vi "(20M)art联动采集V4.9(新增双行扫描模块).vi"() -> ()   [LabVIEW 2016]
uses:
  <vilib>/Utility/file.llb/Write Delimited Spreadsheet (DBL).vi
  E:/PCI8552B/Driver/INF/Win32&Win64/amd64/PCI8552B_32.dll
  <vilib>/Instr/_visa.llb/VISA Configure Serial Port (Instr).vi
  <vilib>/Utility/file.llb/Read Delimited Spreadsheet (I64).vi
  ACTS1001_32.dll
panel:
  in  "输出宽度 3":i32=50 min=50 max=50000 step=50
  in  "输出宽度 2":i32=50 min=50 max=50000 step=50
  out "hDevice":i32=241832032
  out "采样频率":i32=10000 min=1 max=80000000 step=1
  out "使能通道总数":i32
  in  "分频数":i32=20 min=1 step=1
  in  "是否为主设备":bool caption="触发输出使能"
  in  "时钟输出":i32(ring) items=["参考时钟", "基准时钟"]
  in  "时钟输出 2":bool caption="触发输出使能"
  in  "采样时基":i32(ring) items=["内部时钟", "外部时钟"]
  in  "参考时钟":i32(ring) items=["板载时钟", "外部10M", "PXI_CLK10M", "PXIe_CLK100M"]
  in  "输出宽度":i32=50 min=50 max=50000 step=50
  in  "触发输出使能":bool
  in  "触发输出":i32(ring) items=["负向触发", "正向触发", "正负向触发"]
  in  "延时点数":i32 min=0 step=1
  in  "量程选择 3":i32(ring) items=["±5000mV"=0, "±1000mV"=2]
  in  "量程选择 2":i32(ring) items=["±5000mV"=0, "±1000mV"=2]
  in  "量程选择 1":i32(ring) items=["±5000mV"=0, "±1000mV"=2]
  in  "量程选择 0":i32(ring) items=["±5000mV"=0, "±1000mV"=2]
  in  "CH3":bool=TRUE
  in  "CH2":bool=TRUE
  in  "CH1":bool=TRUE
  in  "CH0":bool=TRUE
  in  "耦合类型1":i32(ring) items=["直流", "交流"]
  in  "耦合类型0":i32(ring) items=["直流", "交流"]
  in  "耦合类型2":i32(ring) items=["直流", "交流"]
  in  "耦合类型3":i32(ring) items=["直流", "交流"]
  in  "同步信号触发源":i32(ring) items=["TRIG0信号", "TRIG1信号", "TRIG2信号", "TRIG3信号", "TRIG4信号", "TRIG5信号", "TRIG6信号", "TRIG7信号"]
  in  "触发电平":i32=1 min=1 max=10 step=1
  in  "触发灵敏窗":i32=1 min=1 max=255 step=1
  in  "触发方向":i32(ring) items=["下降沿触发", "上升沿触发", "上升沿下降沿均触发"]
  in  "触发模式":i32(ring) items=["后触发", "硬件延时触发"]
  in  "触发源":i32(ring) items=["软件触发", "外部数字触发", "同步信号触发", "通道0触发", "通道1触发", "通道2触发", "通道3触发"]
  in  "单行？":enum32{"单行", "双行"}(radio)
  in  "色码表导入":path=path "C:/Users/H301/Desktop/art闭环扫描程序/色码表/色码表（彩色2）.txt" caption="（色码表导入）"
  out "水平进度条":u8(slide) scale=0.0..100.0
  out "x+y 3":dbl=3.0
  in  "分层图查看":bool
  in  "hDevice 2":i32
  in  "逐行扫描":bool
  in  "定位模式":bool
  in  "X终点":dbl
  in  "Y终点":dbl
  in  "高级设置":bool
  in  "Y轴回零速度":dbl=15000.0
  in  "X轴回零速度":dbl=15000.0
  in  "细分设置":dbl=8.0
  in  "等待时间":u32=40
  in  "文件保存":path=path "C:/Users/H301/Desktop/art采集实验数据" caption="保存路径"
  out "已用时（s）":dbl format="%<%H:%M:%S>t"
  out "error out":errorcluster caption="错误输出"
  in  "退出扫描(Esc)":bool
  out "毫秒计时值":u32=3586537
  out "数组":dbl[][](array[numeric])=[[58819.77200735986, 88200.32943600747]]
  out "强度图":dbl[][](graph)=[[58819.77200735986, 88200.32943600747]]
  out "judge":dbl
  out "Xloop":dbl
  out "幅频谱":dbl[](graph)
  out "时域谱":dbl[](graph)
  out "错误输出":errorcluster
  in  "启动":bool
  in  "逐点扫描":bool
  in  "X归零":bool
  in  "Y归零":bool
  in  "Y起点":dbl
  in  "Y轴速度":dbl=9000.0
  in  "X轴速度":dbl=9000.0
  out "电机状态":bool
  in  "电机端口":refnum<visa-resource-name>="COM6"
  out "Yloop":dbl=1.0
  out "X扫描范围":dbl=150.0
  out "Y扫描范围":dbl=75.0
  out "Y序":i32
  in  "X起点":dbl
  out "Y(mm)":dbl
  out "x+y 2":dbl=3.0
  in  "Y:":dbl=1.0
  in  "精度":dbl=0.001
  in  "电机急停":bool
  out "X（mm）":dbl
  out "x+y":dbl=1.0
  in  "X:":dbl=1.0
  # "实时坐标"
  # "时域谱"
  # "频域谱"
  # "归零"
  # "扫描区域"
  # "扫描步进(mm)"
  # "X:"
  # "~"
  # "Y:"
  # "~"
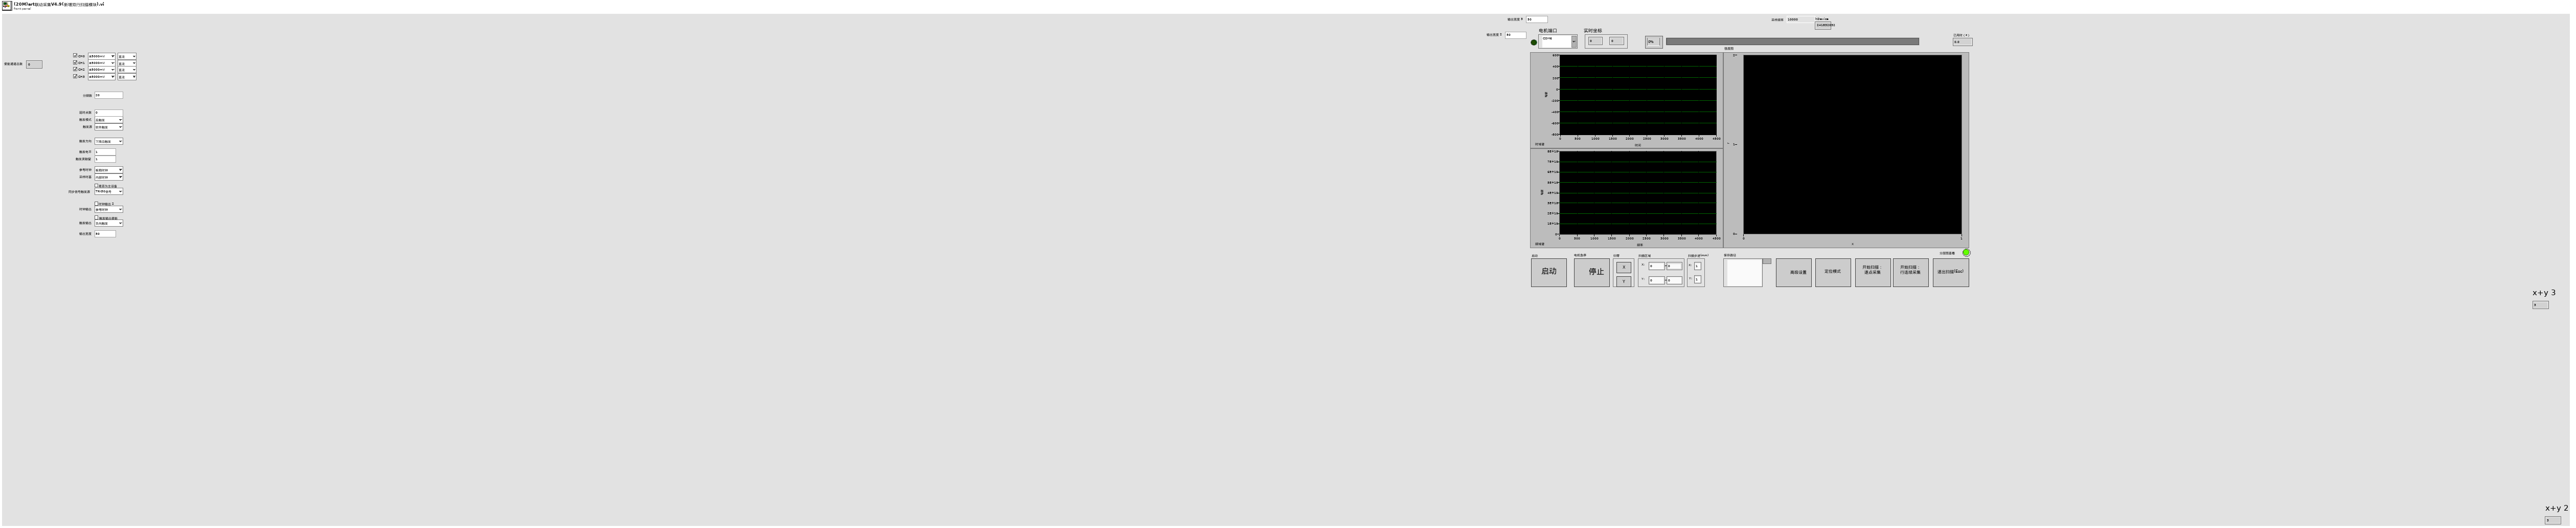
[diagram p1: front panel]
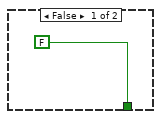
[diagram p2: hidden frame]
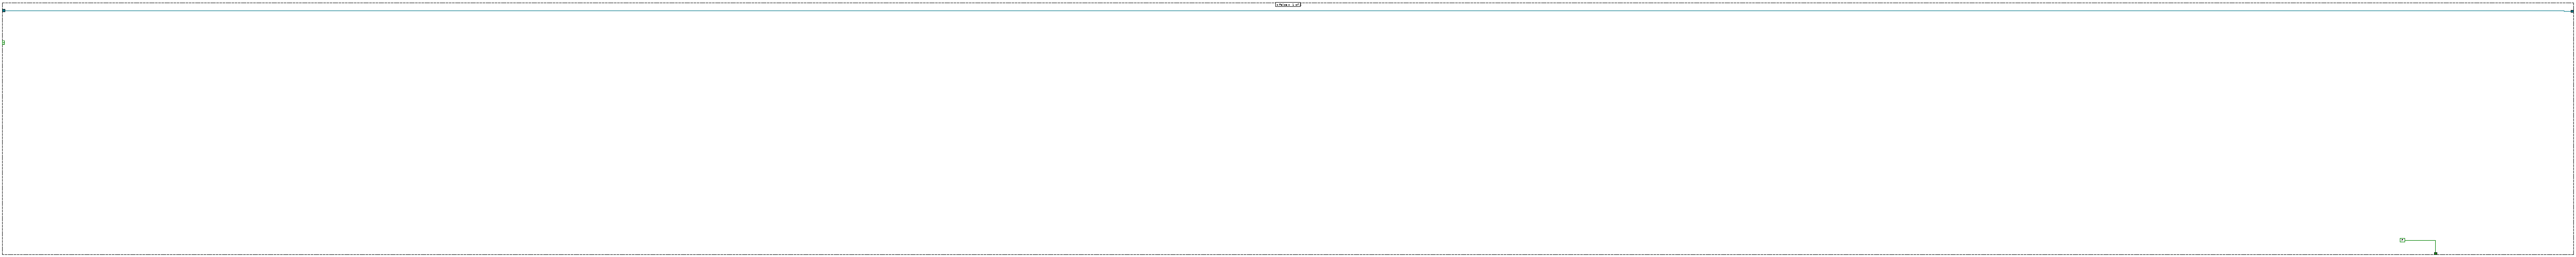
[diagram p3: hidden frame]
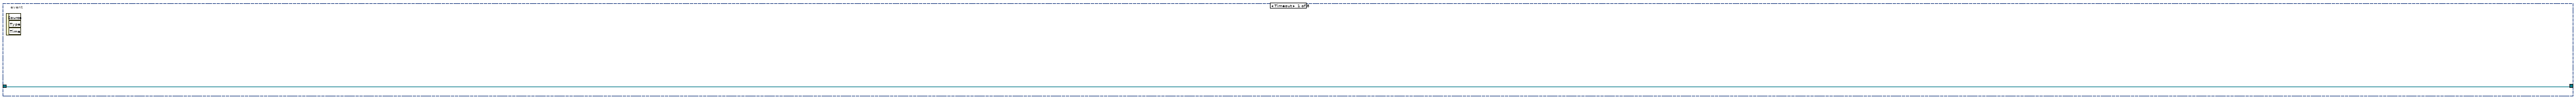
[diagram p4: hidden frame]
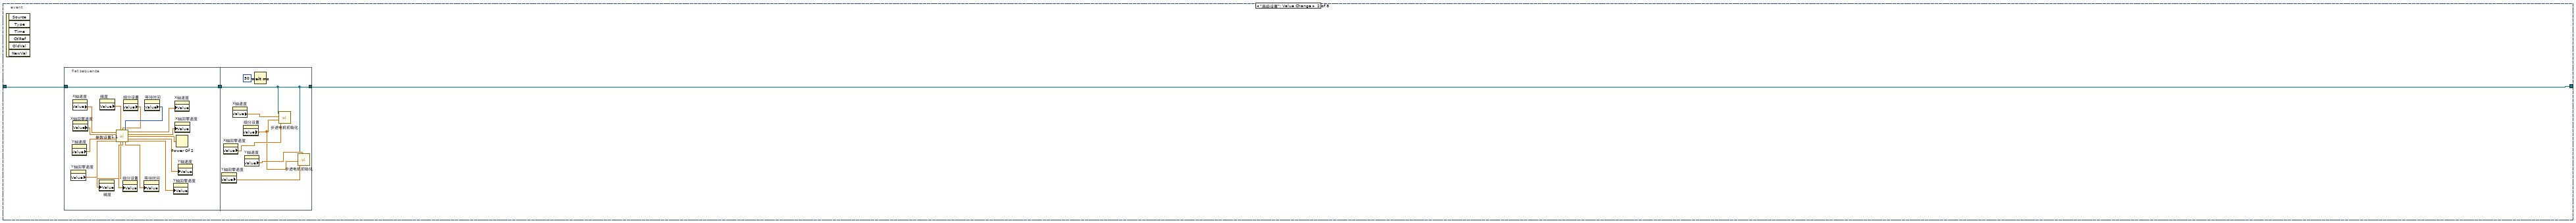
[diagram p5: hidden frame]
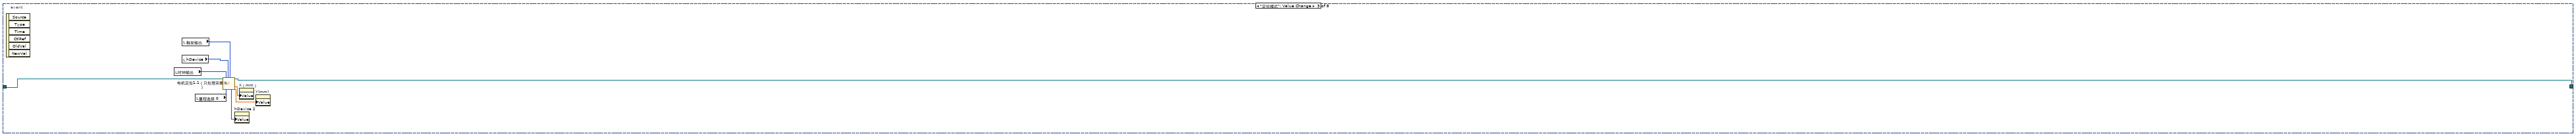
[diagram p6: hidden frame]
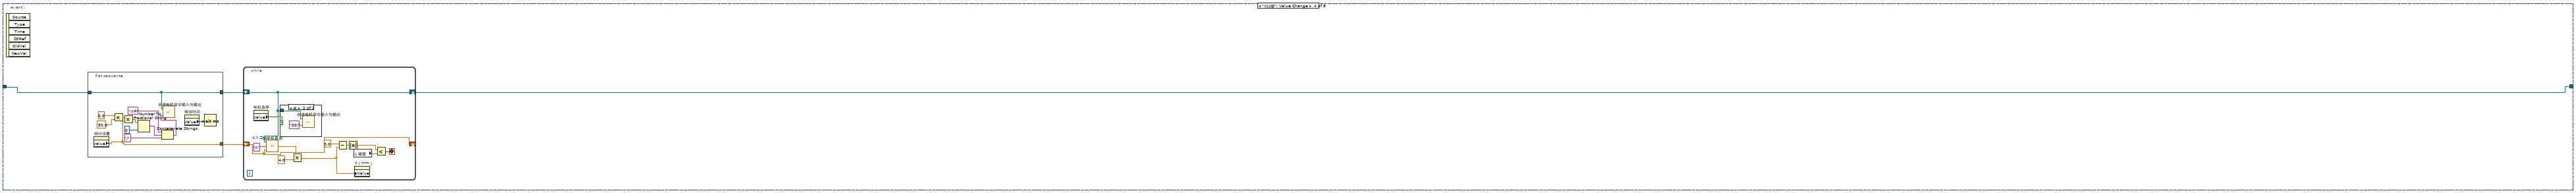
[diagram p7: hidden frame]
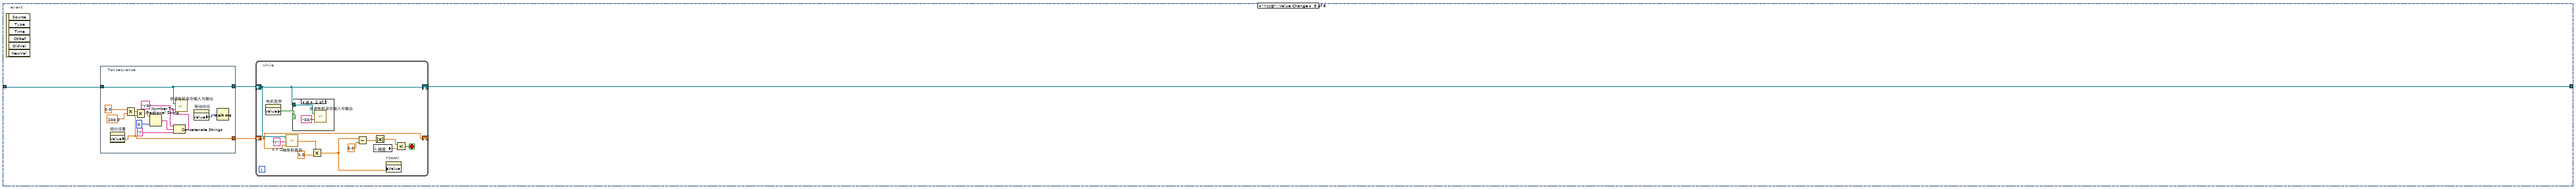
[diagram p9: hidden frame]
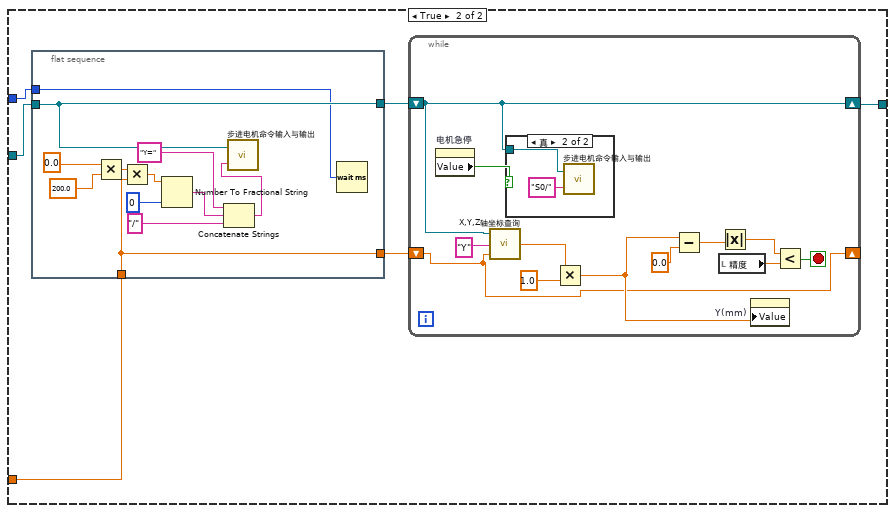
[diagram p15: hidden frame]
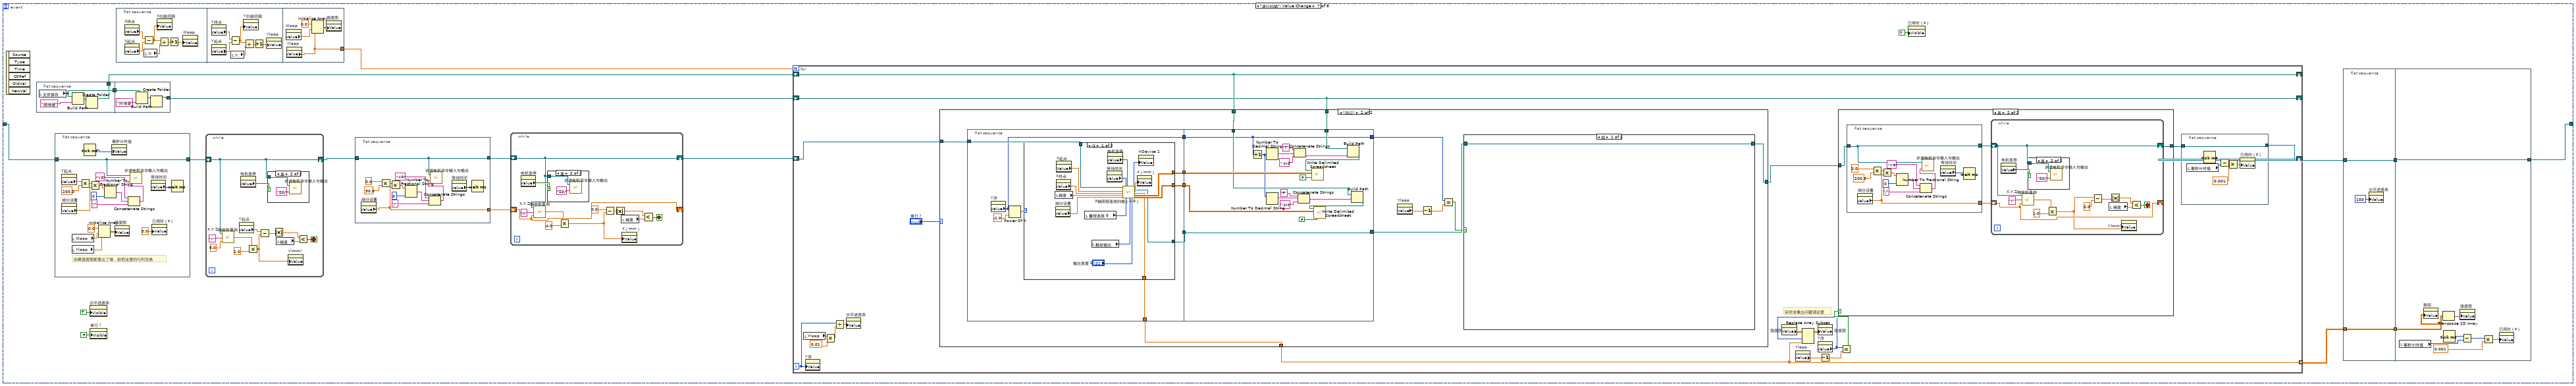
[diagram p19: hidden frame]
diagram:
  n1 = call-poly <vilib>:"Read Delimited Spreadsheet.vi"("file path (dialog if empty)"="色码表导入") -> ("first row"=w2:i64[])  [unwired: 9 in, 5 out]
  n2 = property on="强度图" class="IntGraph (严格)"("Color Table"=w2) -> ()  [unwired: 2 in, 2 out]
  n3 = property on="水平进度条" class="Slide (严格)"("Visible"=FALSE ("可见")) -> ()  [unwired: 2 in, 2 out]
  n4 = property on="单行？" class="RadioBtnsControl (严格)"("Visible"=TRUE ("可见")) -> ()  [unwired: 2 in, 2 out]
  n5 = while {
    stop <- w8 stop-if-true
    n6 = case shown="真" "启动" {
      tunnel: [FALSE ("ESC") w72] -> w8
      frame False {
      }
      frame True {
        w39 = 0 items=["边沿触发", "脉冲触发"] ("触发类型")
        w85 = u16 0 items=["无", "XON/XOFF", "RTS/CTS", "XON/XOFF & RTS/CTS", "DTR/DSR", "XON/XOFF & DTR/DSR"] ("flow control (0:none)")
        w86 = u16 10 items=["1.0"=10, "1.5"=15, "2.0"=20] ("stop bits (10: 1 bit)")
        n7 = local write item#-1(FALSE ("停止")) -> ()
        n8 = Boolean To (0,1)(Boolean="CH0") -> (0, 1=w60:i16)
        n9 = Boolean To (0,1)(Boolean="CH1") -> (0, 1=w59:i16)
        n10 = Boolean To (0,1)(Boolean="CH2") -> (0, 1=w58:i16)
        n11 = Boolean To (0,1)(Boolean="CH3") -> (0, 1=w57:i16)
        n12 = To Long Integer(number=w60) -> (32bit integer=w56:i32)
        n13 = To Long Integer(number=w59) -> (32bit integer=w55:i32)
        n14 = To Long Integer(number=w58) -> (32bit integer=w54:i32)
        n15 = To Long Integer(number=w57) -> (32bit integer=w53:i32)
        n16 = Build Array("耦合类型0", "耦合类型1", "耦合类型2", "耦合类型3") -> (w43:i32[])
        n17 = Build Array(w56, w55, w54, w53) -> (w19:i32[])
        n18 = Build Array("量程选择 0", "量程选择 1", "量程选择 2", "量程选择 3") -> (w48:i32[])
        n19 = Boolean To (0,1)(Boolean="是否为主设备") -> (0, 1=w33:i16)
        n20 = Boolean To (0,1)(Boolean="时钟输出 2") -> (0, 1=w32:i16)
        n21 = dll-call lib="ACTS1001_32.dll" fn="ACTS1001_CreateDevice"("DeviceLgcID"=0) -> ("hDevice"=w13:i32)  [unwired: 4 in, 2 out]
        n22 = Boolean To (0,1)(Boolean="触发输出使能") -> (0, 1=w31:i16)
        n23 = To Long Integer(number=w33) -> (32bit integer=w29:i32)
        n24 = To Long Integer(number=w32) -> (32bit integer=w26:i32)
        n25 = To Long Integer(number=w31) -> (32bit integer=w24:i32)
        n26 = Add Array Elements(numeric array=w19) -> (sum=→"使能通道总数":i32)
        n27 = call-poly "VISA Configure Serial Port"("VISA resource name"="电机端口", "baud rate (9600)"=u32 9600, "data bits (8)"=u16 8, "parity (0:none)"=enum16{"None", "Odd", "Even", "Mark", "Space"}."None", "stop bits (10: 1 bit)"=w86, "flow control (0:none)"=w85) -> ("VISA resource name out"=w77:refnum<visa-resource-name>, "error out"=→"error out":errorcluster)  [unwired: 1 in, 7 out]
        n28 = Build Array (concatenate)(w19, w48, w43, "分频数", "延时点数", "触发模式", "触发源", w39, "触发方向", "触发电平", "触发灵敏窗", "参考时钟", "采样时基", w29, "同步信号触发源", w26, "时钟输出", w24, "触发输出", "输出宽度") -> (w12:i32[])
        n29 = Divide(x=40000000, y="分频数") -> (x/y=→"采样频率":dbl)
        n30 = property on="细分设置" class="DigNum (严格)"() -> ("Value"=w71:dbl)  [unwired: 2 in, 2 out]
        n31 = call "步进电机初始化.vi"("回零速度"="X轴回零速度", "细分设置"=w71, "X轴速度"="X轴速度", "串口通信端口"=w77) -> ()  [unwired: 2 in, 1 out]
        n32 = call "步进电机初始化.vi"("Y轴速度"="Y轴速度", "回零速度"="Y轴回零速度", "细分设置"=w71, "串口通信端口"=w77) -> ()  [unwired: 2 in, 1 out]
        n33 = dll-call lib="ACTS1001_32.dll" fn="ACTS1001_InitDeviceAD"("hDevice"=w13, "pADPara"=w12) -> ("hDevice"=→"hDevice":i32)  [unwired: 5 in, 2 out]
        n34 = call "步进电机命令输入与输出.vi"("输入字符串"="?R/", "串口通信端口"=w77) -> ("返回字符串"=w82:string)
        n35 = String Subset(string=w82, offset (0)=0 ("偏移量(0)"), length (rest)=2 ("长度（剩余）")) -> (substring=w79:string)
        n36 = Equal?(x=w79, y="OK") -> (x = y?=w76:bool)
        "电机状态" <- w76
        n37 = case shown="真" w76 {
          tunnel: w77 -> [w92 w95]
          tunnel: [w92 w93] -> w73
          tunnel: [FALSE ("ESC") w94] -> w72
          frame False {
          }
          frame True {
            n38 = while {
              tunnel: ["退出扫描(Esc)"] -> w94
              shift-right: [w99] -> w93
              shift-left: w95 -> [w104]
              stop <- "退出扫描(Esc)" stop-if-true
              n39 = property on="水平进度条" class="Slide (严格)"("Visible"=FALSE ("可见")) -> ()  [unwired: 2 in, 2 out]
              n40 = property on="高级设置" class="Bool"("Visible"=TRUE ("可见")) -> ()  [unwired: 2 in, 2 out]
              n41 = property on="定位模式" class="Bool"("Visible"=TRUE ("可见")) -> ()  [unwired: 2 in, 2 out]
              n42 = property on="水平进度条" class="Slide (严格)"("Value"=u8 0 ("水平进度条")) -> ()  [unwired: 2 in, 2 out]
              n43 = property on="单行？" class="RadioBtnsControl (严格)"("Visible"=TRUE ("可见")) -> ()  [unwired: 2 in, 2 out]
              n44 = event shown="[5] \"逐点扫描\": 值改变" {
                selector: _ -> [_ _ _ _ _ _ _ _]
                dyn-events: _ -> [_ _ _ _ _ _ _ _]
                timeout: 1 -> [_ _ _ _ _ _ _ _]
                tunnel: w104 -> [w105 w108 w141 w145 w175 w226 w540 w905]
                tunnel: [w105 w107 w140 w143 w173 w221 w542 w904] -> w99
                event Timeout {
                  n45 = event-data() -> ()  [unwired: 1 in, 3 out]
                }
                event "高级设置": Value Change {
                  n46 = event-data() -> ()  [unwired: 1 in, 6 out]
                  n47 = flat-sequence {
                    tunnel: w108 -> [w111]
                    tunnel: [w111] -> w106
                    tunnel: [w127] -> w107
                    tunnel: w106 -> [w127]
                    frame #0 {
                      n48 = property on="Y轴回零速度" class="DigNum (严格)"() -> ("Value"=w115:dbl)  [unwired: 2 in, 2 out]
                      n49 = property on="Y轴速度" class="DigNum (严格)"() -> ("Value"=w114:dbl)  [unwired: 2 in, 2 out]
                      n50 = property on="X轴速度" class="DigNum (严格)"() -> ("Value"=w112:dbl)  [unwired: 2 in, 2 out]
                      n51 = property on="X轴回零速度" class="DigNum (严格)"() -> ("Value"=w113:dbl)  [unwired: 2 in, 2 out]
                      n52 = property on="精度" class="DigNum (严格)"() -> ("Value"=w119:dbl)  [unwired: 2 in, 2 out]
                      n53 = property on="细分设置" class="DigNum (严格)"() -> ("Value"=w120:dbl)  [unwired: 2 in, 2 out]
                      n54 = property on="等待时间" class="DigNum (严格)"() -> ("Value"=w121:u32)  [unwired: 2 in, 2 out]
                      n55 = call "参数设置1.1.vi"("X轴速度"=w112, "精度"=w119, "细分设置"=w120, "等待时间"=w121, "X轴回零速度"=w113, "Y轴速度"=w114, "Y轴回零速度"=w115) -> ("X轴速度"=w122:dbl, "X轴回零速度"=w123:dbl, "采样阶"=w109:dbl, "Y轴速度"=w124:dbl, "精度"=w116:dbl, "细分设置"=w117:dbl, "等待时间"=w118:dbl, "Y轴回零速度"=w125:dbl)  [unwired: 1 in]
                      n56 = property on="精度" class="DigNum (严格)"("Value"=w116) -> ()  [unwired: 2 in, 2 out]
                      n57 = property on="细分设置" class="DigNum (严格)"("Value"=w117) -> ()  [unwired: 2 in, 2 out]
                      n58 = property on="等待时间" class="DigNum (严格)"("Value"=w118) -> ()  [unwired: 2 in, 2 out]
                      n59 = property on="Y轴回零速度" class="DigNum (严格)"("Value"=w125) -> ()  [unwired: 2 in, 2 out]
                      n60 = property on="X轴速度" class="DigNum (严格)"("Value"=w122) -> ()  [unwired: 2 in, 2 out]
                      n61 = property on="X轴回零速度" class="DigNum (严格)"("Value"=w123) -> ()  [unwired: 2 in, 2 out]
                      n62 = Power Of 2(x=w109) -> (2^x=w110:dbl)
                      n63 = property on="Y轴速度" class="DigNum (严格)"("Value"=w124) -> ()  [unwired: 2 in, 2 out]
                    }
                    frame #1 {
                      n64 = property on="Y轴回零速度" class="DigNum (严格)"() -> ("Value"=w131:dbl)  [unwired: 2 in, 2 out]
                      n65 = property on="X轴回零速度" class="DigNum (严格)"() -> ("Value"=w130:dbl)  [unwired: 2 in, 2 out]
                      n66 = property on="X轴速度" class="DigNum (严格)"() -> ("Value"=w129:dbl)  [unwired: 2 in, 2 out]
                      n67 = property on="细分设置" class="DigNum (严格)"() -> ("Value"=w128:dbl)  [unwired: 2 in, 2 out]
                      n68 = property on="Y轴速度" class="DigNum (严格)"() -> ("Value"=w132:dbl)  [unwired: 2 in, 2 out]
                      n69 = Wait (ms)(milliseconds to wait=u32 50 ("等待时间（毫秒）")) -> ()  [unwired: 1 out]
                      n70 = call "步进电机初始化.vi"("回零速度"=w130, "细分设置"=w128, "X轴速度"=w129, "串口通信端口"=w127) -> ()  [unwired: 2 in, 1 out]
                      n71 = call "步进电机初始化.vi"("Y轴速度"=w132, "回零速度"=w131, "细分设置"=w128, "串口通信端口"=w127) -> ()  [unwired: 2 in, 1 out]
                    }
                  }
                }
                event "定位模式": Value Change {
                  n72 = event-data() -> ()  [unwired: 1 in, 6 out]
                  n73 = local read "时钟输出"() -> (w137:i32)
                  n74 = local read "触发输出"() -> (w136:i32)
                  n75 = local read "hDevice"() -> (w133:i32)
                  n76 = local read "量程选择 0"() -> (w134:i32)
                  n77 = call "电机定位1.1（只处理采集卡）.vi"("VISA I"=w141, "pulDDR2Length"=w137, "量程选择"=w134, "hDevice"=w133, "M-length"=w136) -> ("hDevice out"=w135:i32, "VISA O"=w140:refnum<visa-resource-name>, "X"=w139:dbl, "Y"=w138:dbl)  [unwired: 11 in]
                  n78 = property on="hDevice 2" class="DigNum (严格)"("Value"=w135) -> ()  [unwired: 2 in, 2 out]
                  n79 = property on="X（mm）" class="DigNum (严格)"("Value"=w139) -> ()  [unwired: 2 in, 2 out]
                  n80 = property on="Y(mm)" class="DigNum (严格)"("Value"=w138) -> ()  [unwired: 2 in, 2 out]
                }
                event "X归零": Value Change {
                  n81 = event-data() -> ()  [unwired: 1 in, 6 out]
                  n82 = flat-sequence {
                    tunnel: w145 -> [w149]
                    tunnel: [w149] -> w144
                    tunnel: [w146] -> w142
                    frame #0 {
                      n83 = property on="细分设置" class="DigNum (严格)"() -> ("Value"=w146:dbl)  [unwired: 2 in, 2 out]
                      n84 = Multiply(x=0.0, y=50.0) -> (x*y=w152:dbl)
                      n85 = Multiply(x=w152, y=w146) -> (x*y=w157:dbl)
                      n86 = Number To Fractional String(number=w157, precision (6)=i16 0 ("精度(6)")) -> (F-format string=w155:string)  [unwired: 2 out]
                      n87 = Concatenate Strings("X=" ("字符串"), w155, "/" ("字符串")) -> (w150:string)
                      n88 = call "步进电机命令输入与输出.vi"("输入字符串"=w150, "串口通信端口"=w149) -> ()  [unwired: 1 out]
                      n89 = property on="等待时间" class="DigNum (严格)"() -> ("Value"=w147:u32)  [unwired: 2 in, 2 out]
                      n90 = Wait (ms)(milliseconds to wait=w147) -> ()  [unwired: 1 out]
                    }
                  }
                  n91 = while {
                    shift-right: [w159] -> w143
                    shift-left: w144 -> [w159]
                    shift-right: [w158] -> _
                    shift-left: w142 -> [w158]
                    stop <- w165 stop-if-true
                    n92 = property on="电机急停" class="Bool (严格)"() -> ("Value"=w166:bool)  [unwired: 2 in, 2 out]
                    n93 = call "X,Y,Z轴坐标查询.vi"("细分设置"=w158, "查询坐标轴"="X", "串口通信端口"=w159) -> ("坐标(mm)"=w167:dbl)
                    n94 = case shown="真" w166 {
                      tunnel: w159 -> [_ w170]
                      frame False {
                      }
                      frame True {
                        n95 = call "步进电机命令输入与输出.vi"("输入字符串"="S0/", "串口通信端口"=w170) -> ()  [unwired: 1 out]
                      }
                    }
                    n96 = Multiply(x=w167, y=4.0 ("x")) -> (x*y=w163:dbl)
                    n97 = Subtract(x=0.0, y=w163) -> (x-y=w162:dbl)
                    n98 = Absolute Value(x=w162) -> (abs(x)=w161:dbl)
                    n99 = local read "精度"() -> (w164:dbl)
                    n100 = property on="X（mm）" class="DigNum (严格)"("Value"=w163) -> ()  [unwired: 2 in, 2 out]
                    n101 = Less?(x=w161, y=w164) -> (x < y?=w165:bool)
                  }
                }
                event "Y归零": Value Change {
                  n102 = event-data() -> ()  [unwired: 1 in, 6 out]
                  n103 = flat-sequence {
                    tunnel: w175 -> [w179]
                    tunnel: [w179] -> w174
                    tunnel: [w176] -> w172
                    frame #0 {
                      n104 = property on="细分设置" class="DigNum (严格)"() -> ("Value"=w176:dbl)  [unwired: 2 in, 2 out]
                      n105 = Multiply(x=0.0, y=200.0) -> (x*y=w182:dbl)
                      n106 = Multiply(x=w182, y=w176) -> (x*y=w187:dbl)
                      n107 = Number To Fractional String(number=w187, precision (6)=i16 0 ("精度(6)")) -> (F-format string=w185:string)  [unwired: 2 out]
                      n108 = Concatenate Strings("Y=" ("字符串"), w185, "/" ("字符串")) -> (w180:string)
                      n109 = call "步进电机命令输入与输出.vi"("输入字符串"=w180, "串口通信端口"=w179) -> ()  [unwired: 1 out]
                      n110 = property on="等待时间" class="DigNum (严格)"() -> ("Value"=w177:u32)  [unwired: 2 in, 2 out]
                      n111 = Wait (ms)(milliseconds to wait=w177) -> ()  [unwired: 1 out]
                    }
                  }
                  n112 = while {
                    shift-right: [w189] -> w173
                    shift-left: w174 -> [w189]
                    shift-right: [w188] -> _
                    shift-left: w172 -> [w188]
                    stop <- w195 stop-if-true
                    n113 = property on="电机急停" class="Bool (严格)"() -> ("Value"=w196:bool)  [unwired: 2 in, 2 out]
                    n114 = call "X,Y,Z轴坐标查询.vi"("细分设置"=w188, "查询坐标轴"="Y", "串口通信端口"=w189) -> ("坐标(mm)"=w197:dbl)
                    n115 = case shown="真" w196 {
                      tunnel: w189 -> [_ w200]
                      frame False {
                      }
                      frame True {
                        n116 = call "步进电机命令输入与输出.vi"("输入字符串"="S0/", "串口通信端口"=w200) -> ()  [unwired: 1 out]
                      }
                    }
                    n117 = Multiply(x=w197, y=1.0 ("x")) -> (x*y=w193:dbl)
                    n118 = Subtract(x=w193, y=0.0 ("x")) -> (x-y=w191:dbl)
                    n119 = local read "精度"() -> (w194:dbl)
                    n120 = Absolute Value(x=w191) -> (abs(x)=w190:dbl)
                    n121 = property on="Y(mm)" class="DigNum (严格)"("Value"=w193) -> ()  [unwired: 2 in, 2 out]
                    n122 = Less?(x=w190, y=w194) -> (x < y?=w195:bool)
                  }
                }
                event "逐点扫描": Value Change {
                  n123 = event-data() -> ()  [unwired: 1 in, 6 out]
                  n124 = flat-sequence {
                    tunnel: w226 -> [w255]
                    tunnel: [w255] -> w217
                    frame #0 {
                      # "如果强度图那里出了错，就把这里的行列互换"
                      n125 = Tick Count (ms)() -> (millisecond timer value=→"毫秒计时值":u32)
                      n126 = local read "Xloop"() -> (w250:dbl)
                      n127 = local read "Yloop"() -> (w249:dbl)
                      n128 = Multiply(x="Y起点", y=200.0) -> (x*y=w258:dbl)
                      n129 = Multiply(x=w258, y="细分设置") -> (x*y=w263:dbl)
                      n130 = Initialize Array(0.0 ("元素"), w250, w249) -> (→"强度图":dbl[][])
                      n131 = Number To Fractional String(number=w263, precision (6)=i16 0 ("精度(6)")) -> (F-format string=w261:string)  [unwired: 2 out]
                      n132 = Concatenate Strings("Y=" ("字符串"), w261, "/" ("字符串")) -> (w256:string)
                      n133 = call "步进电机命令输入与输出.vi"("输入字符串"=w256, "串口通信端口"=w255) -> ()  [unwired: 1 out]
                      n134 = property on="已用时（s）" class="DigNum (严格)"("Value"=0.0 ("已用时（s）")) -> ()  [unwired: 2 in, 2 out]
                      n135 = property on="等待时间" class="DigNum (严格)"() -> ("Value"=w247:u32)  [unwired: 2 in, 2 out]
                      n136 = Wait (ms)(milliseconds to wait=w247) -> ()  [unwired: 1 out]
                    }
                  }
                  n137 = local read "X起点"() -> (w213:dbl)
                  n138 = property on="水平进度条" class="Slide (严格)"("Visible"=TRUE ("可见")) -> ()  [unwired: 2 in, 2 out]
                  n139 = Subtract(x="X终点", y=w213) -> (x-y=w212:dbl)
                  "X扫描范围" <- w212
                  n140 = local read "X:"() -> (w220:dbl)
                  n141 = Divide(x=w212, y=w220) -> (x/y=w218:dbl)
                  n142 = Increment(x=w218) -> (x+1=→"Xloop":dbl)
                  n143 = while {
                    shift-right: [w264] -> w209
                    shift-left: w217 -> [w264]
                    stop <- w269 stop-if-true
                    n144 = call "X,Y,Z轴坐标查询.vi"("细分设置"=8.0, "查询坐标轴"="Y", "串口通信端口"=w264) -> ("坐标(mm)"=w271:dbl)
                    n145 = property on="Y起点" class="DigNum (严格)"() -> ("Value"=w273:dbl)  [unwired: 2 in, 2 out]
                    n146 = property on="电机急停" class="Bool (严格)"() -> ("Value"=w270:bool)  [unwired: 2 in, 2 out]
                    n147 = Multiply(x=w271, y=1.0 ("x")) -> (x*y=w267:dbl)
                    n148 = Subtract(x=w273, y=w267) -> (x-y=w266:dbl)
                    n149 = case shown="真" w270 {
                      tunnel: w264 -> [_ w276]
                      frame False {
                      }
                      frame True {
                        n150 = call "步进电机命令输入与输出.vi"("输入字符串"="S0/", "串口通信端口"=w276) -> ()  [unwired: 1 out]
                      }
                    }
                    n151 = Absolute Value(x=w266) -> (abs(x)=w265:dbl)
                    n152 = local read "精度"() -> (w268:dbl)
                    n153 = property on="Y(mm)" class="DigNum (严格)"("Value"=w267) -> ()  [unwired: 2 in, 2 out]
                    n154 = Less?(x=w265, y=w268) -> (x < y?=w269:bool)
                  }
                  n155 = local read "Y起点"() -> (w215:dbl)
                  n156 = Subtract(x="Y终点", y=w215) -> (x-y=w211:dbl)
                  "Y扫描范围" <- w211
                  n157 = local read "Y:"() -> (w225:dbl)
                  n158 = Divide(x=w211, y=w225) -> (x/y=w224:dbl)
                  n159 = Increment(x=w224) -> (x+1=w223:dbl)
                  "Yloop" <- w223
                  n160 = for {
                    N: w223 -> [_]
                    shift-right: [w301] -> w202
                    shift-left: w209 -> [w282]
                    tunnel: [w284] -> w222 mode=indexing
                    tunnel: w207 -> [w288]
                    tunnel: w210 -> [w287]
                    i -> [w302]
                    # "实时成像出问题调这里"
                    n161 = flat-sequence {
                      tunnel: w282 -> [w359]
                      tunnel: [w359] -> w300
                      tunnel: [w358] -> w292
                      frame #0 {
                        n162 = property on="X起点" class="DigNum (严格)"() -> ("Value"=w356:dbl)  [unwired: 2 in, 2 out]
                        n163 = property on="细分设置" class="DigNum (严格)"() -> ("Value"=w358:dbl)  [unwired: 2 in, 2 out]
                        n164 = local read "等待时间"() -> (w357:u32)
                        n165 = Multiply(x=w356, y=50.0) -> (x*y=w362:dbl)
                        n166 = Multiply(x=w362, y=w358) -> (x*y=w367:dbl)
                        n167 = Wait (ms)(milliseconds to wait=w357) -> ()  [unwired: 1 out]
                        n168 = Number To Fractional String(number=w367, precision (6)=i16 0 ("精度(6)")) -> (F-format string=w365:string)  [unwired: 2 out]
                        n169 = Concatenate Strings("X=" ("字符串"), w365, "/" ("字符串")) -> (w360:string)
                        n170 = call "步进电机命令输入与输出.vi"("输入字符串"=w360, "串口通信端口"=w359) -> ()  [unwired: 1 out]
                      }
                    }
                    n171 = while {
                      shift-right: [w369] -> w280
                      shift-left: w300 -> [w369]
                      shift-right: [w368] -> _
                      shift-left: w292 -> [w368]
                      stop <- w374 stop-if-true
                      n172 = property on="电机急停" class="Bool (严格)"() -> ("Value"=w375:bool)  [unwired: 2 in, 2 out]
                      n173 = case shown="真" w375 {
                        tunnel: w369 -> [_ w380]
                        frame False {
                        }
                        frame True {
                          n174 = call "步进电机命令输入与输出.vi"("输入字符串"="S0/", "串口通信端口"=w380) -> ()  [unwired: 1 out]
                        }
                      }
                      n175 = call "X,Y,Z轴坐标查询.vi"("细分设置"=w368, "查询坐标轴"="X", "串口通信端口"=w369) -> ("坐标(mm)"=w376:dbl)
                      n176 = Multiply(x=w376, y=4.0 ("x")) -> (x*y=w372:dbl)
                      n177 = property on="X起点" class="DigNum (严格)"() -> ("Value"=w378:dbl)  [unwired: 2 in, 2 out]
                      n178 = Subtract(x=w378, y=w372) -> (x-y=w371:dbl)
                      n179 = Absolute Value(x=w371) -> (abs(x)=w370:dbl)
                      n180 = local read "精度"() -> (w373:dbl)
                      n181 = property on="X（mm）" class="DigNum (严格)"("Value"=w372) -> ()  [unwired: 2 in, 2 out]
                      n182 = Less?(x=w370, y=w373) -> (x < y?=w374:bool)
                    }
                    n183 = local read "Xloop"() -> (w293:dbl)
                    n184 = for {
                      N: w293 -> [_]
                      shift-right: [w463] -> w281
                      shift-left: w280 -> [w459]
                      tunnel: [w462] -> w299 mode=indexing
                      tunnel: [w461] -> w298 mode=indexing
                      tunnel: [w460] -> w284 mode=indexing
                      i -> [w451]
                      n185 = flat-sequence {
                        tunnel: w459 -> [w468]
                        tunnel: [w467] -> w464
                        tunnel: w451 -> [w465]
                        tunnel: [w526] -> w463
                        tunnel: w464 -> [w526]
                        tunnel: [w525] -> w462
                        tunnel: [w524] -> w461
                        tunnel: [w522] -> w460
                        frame #0 {
                          n186 = Equal To 0?(x=w465) -> (x = 0?=w466:bool)
                          n187 = case shown="假" w466 {
                            tunnel: w468 -> [w471 w506]
                            tunnel: [w470 w506] -> w467
                            frame False {
                              n188 = flat-sequence {
                                tunnel: w471 -> [w481]
                                tunnel: [w481] -> w472
                                tunnel: [w473] -> w469
                                frame #0 {
                                n189 = local read "X:"() -> (w475:dbl)
                                n190 = Multiply(x=w475, y=1.0 ("x")) -> (x*y=w480:dbl)
                                n191 = property on="等待时间" class="DigNum (严格)"() -> ("Value"=w474:u32)  [unwired: 2 in, 2 out]
                                n192 = property on="细分设置" class="DigNum (严格)"() -> ("Value"=w473:dbl)  [unwired: 2 in, 2 out]
                                n193 = call "X,Y,Z轴坐标查询.vi"("细分设置"=w473, "查询坐标轴"="X", "串口通信端口"=w481) -> ("坐标(mm)"=w477:dbl)
                                n194 = Multiply(x=4.0, y=w477) -> (x*y=w476:dbl)
                                n195 = Add(x=w476, y=w480) -> (x+y=w483:dbl)
                                "x+y" <- w483
                                n196 = Multiply(x=w483, y=50.0) -> (x*y=w486:dbl)
                                n197 = Multiply(x=w486, y=w473) -> (x*y=w491:dbl)
                                n198 = Number To Fractional String(number=w491, precision (6)=i16 0 ("精度(6)")) -> (F-format string=w489:string)  [unwired: 2 out]
                                n199 = Concatenate Strings("X=" ("字符串"), w489, "/" ("字符串")) -> (w484:string)
                                n200 = call "步进电机命令输入与输出.vi"("输入字符串"=w484, "串口通信端口"=w481) -> ()  [unwired: 1 out]
                                n201 = Wait (ms)(milliseconds to wait=w474) -> ()  [unwired: 1 out]
                                }
                              }
                              n202 = while {
                                shift-right: [w501] -> w470
                                shift-left: w472 -> [w501]
                                shift-right: [w492] -> _
                                shift-left: w469 -> [w492]
                                stop <- w500 stop-if-true
                                n203 = property on="电机急停" class="Bool (严格)"() -> ("Value"=w498:bool)  [unwired: 2 in, 2 out]
                                n204 = local read "x+y"() -> (w502:dbl)
                                n205 = case shown="真" w498 {
                                tunnel: w501 -> [_ w504]
                                frame False {
                                }
                                frame True {
                                n206 = call "步进电机命令输入与输出.vi"("输入字符串"="S0/", "串口通信端口"=w504) -> ()  [unwired: 1 out]
                                }
                                }
                                n207 = call "X,Y,Z轴坐标查询.vi"("细分设置"=w492, "查询坐标轴"="X", "串口通信端口"=w501) -> ("坐标(mm)"=w496:dbl)
                                n208 = Multiply(x=4.0, y=w496) -> (x*y=w495:dbl)
                                n209 = Subtract(x=w502, y=w495) -> (x-y=w494:dbl)
                                n210 = property on="X（mm）" class="DigNum (严格)"("Value"=w495) -> ()  [unwired: 2 in, 2 out]
                                n211 = Absolute Value(x=w494) -> (abs(x)=w493:dbl)
                                n212 = local read "精度"() -> (w497:dbl)
                                n213 = Less?(x=w493, y=w497) -> (x < y?=w500:bool)
                              }
                            }
                            frame True {
                            }
                          }
                        }
                        frame #1 {
                          n214 = local read item#-1() -> (w520)
                          n215 = local read item#-1() -> (w521)
                          n216 = call "AD（V3.2）.vi"("M-length"=w520, 11:w521) -> ("幅频谱"=w524:dbl[], "时域谱"=w525:dbl[], "hDevice out"=w508:i32, "N-length"=w509:dbl, "hDevice"=w507:i32)  [unwired: 5 in]
                          "时域谱" <- w525
                          "幅频谱" <- w524
                          n217 = Subtract(x=w509, y=w520) -> (x-y=w518:dbl)
                          n218 = Multiply(x=w518, y=0.25) -> (x*y=w511:dbl)
                          n219 = Multiply(x=w511, y=0.442) -> (x*y=w513:dbl)
                          n220 = Multiply(x=w511, y=0.058) -> (x*y=w515:dbl)
                          n221 = Round Toward -Infinity(1:w513) -> (0:w510:dbl)
                          n222 = Round Toward -Infinity(1:w515) -> (0:w514:dbl)
                          n223 = Increment(x=w510) -> (x+1=w517:dbl)
                          n224 = property on="hDevice 2" class="DigNum (严格)"("Value"=w508) -> ()  [unwired: 2 in, 2 out]
                          n225 = Array Subset(array=w524, index=w514, length=w517) -> (w523:dbl[])
                          n226 = Array Max & Min(array=w523) -> (max value=w522:dbl)  [unwired: 3 out]
                        }
                      }
                      n227 = local read "Y序"() -> (w453:i32)
                      n228 = local read "Xloop"() -> (w454:dbl)
                      n229 = Multiply(x=w453, y=w454) -> (x*y=w452:dbl)
                      n230 = Add(x=w451, y=w452) -> (x+y=w450:dbl)
                      n231 = Multiply(x=w450, y=100.0) -> (x*y=w448:dbl)
                      n232 = local read "Xloop"() -> (w458:dbl)
                      n233 = local read "Yloop"() -> (w457:dbl)
                      n234 = Multiply(x=w457, y=w458) -> (x*y=w456:dbl)
                      n235 = Divide(x=w448, y=w456) -> (x/y=→"水平进度条":dbl)
                    }
                    n236 = flat-sequence {
                      tunnel: w298 -> [w342]
                      tunnel: w299 -> [w350]
                      tunnel: w281 -> [w354]
                      tunnel: [w354] -> w294
                      tunnel: w288 -> [w337]
                      tunnel: w287 -> [w336]
                      frame #0 {
                        n237 = local read "Y序"() -> (w338:i32)
                        n238 = Increment(x=w338) -> (x+1=w339:i32)
                        n239 = Number To Decimal String(number=w339) -> (decimal integer string=w348:string)  [unwired: 1 in]
                        n240 = Number To Decimal String(number=w339) -> (decimal integer string=w347:string)  [unwired: 1 in]
                        n241 = Concatenate Strings("T" ("字符串"), w348, ".txt" ("字符串")) -> (w351:string)
                        n242 = Concatenate Strings("F" ("字符串"), w347, ".txt" ("字符串")) -> (w345:string)
                        n243 = Build Path(base path=w337, name or relative path=w351) -> (appended path=w353:path)
                        n244 = call-poly <vilib>:"Write Delimited Spreadsheet.vi"("file path (dialog if empty)"=w353, "2D data"=w350, "transpose? (no:F)"=FALSE) -> ()  [unwired: 11 in, 2 out]
                        n245 = Build Path(base path=w336, name or relative path=w345) -> (appended path=w343:path)
                        n246 = call-poly <vilib>:"Write Delimited Spreadsheet.vi"("file path (dialog if empty)"=w343, "2D data"=w342, "transpose? (no:F)"=FALSE) -> ()  [unwired: 11 in, 2 out]
                        "judge" <- 1.0
                      }
                    }
                    n247 = flat-sequence {
                      tunnel: w294 -> [w313]
                      tunnel: [w313] -> w295
                      tunnel: [w311] -> w291
                      frame #0 {
                        n248 = property on="细分设置" class="DigNum (严格)"() -> ("Value"=w311:dbl)  [unwired: 2 in, 2 out]
                        n249 = property on="等待时间" class="DigNum (严格)"() -> ("Value"=w310:u32)  [unwired: 2 in, 2 out]
                        n250 = Multiply(x=0.0, y=50.0) -> (x*y=w316:dbl)
                        n251 = Multiply(x=w316, y=w311) -> (x*y=w321:dbl)
                        n252 = Wait (ms)(milliseconds to wait=w310) -> ()  [unwired: 1 out]
                        n253 = Number To Fractional String(number=w321, precision (6)=i16 0 ("精度(6)")) -> (F-format string=w319:string)  [unwired: 2 out]
                        n254 = Concatenate Strings("X=" ("字符串"), w319, "/" ("字符串")) -> (w314:string)
                        n255 = call "步进电机命令输入与输出.vi"("输入字符串"=w314, "串口通信端口"=w313) -> ()  [unwired: 1 out]
                      }
                    }
                    n256 = while {
                      shift-right: [w323] -> w279
                      shift-left: w295 -> [w323]
                      shift-right: [w322] -> _
                      shift-left: w291 -> [w322]
                      stop <- w329 stop-if-true
                      n257 = property on="电机急停" class="Bool (严格)"() -> ("Value"=w330:bool)  [unwired: 2 in, 2 out]
                      n258 = call "X,Y,Z轴坐标查询.vi"("细分设置"=w322, "查询坐标轴"="X", "串口通信端口"=w323) -> ("坐标(mm)"=w331:dbl)
                      n259 = case shown="真" w330 {
                        tunnel: w323 -> [_ w334]
                        frame False {
                        }
                        frame True {
                          n260 = call "步进电机命令输入与输出.vi"("输入字符串"="S0/", "串口通信端口"=w334) -> ()  [unwired: 1 out]
                        }
                      }
                      n261 = Multiply(x=w331, y=4.0 ("x")) -> (x*y=w327:dbl)
                      n262 = Subtract(x=0.0, y=w327) -> (x-y=w326:dbl)
                      n263 = Absolute Value(x=w326) -> (abs(x)=w325:dbl)
                      n264 = local read "精度"() -> (w328:dbl)
                      n265 = property on="X（mm）" class="DigNum (严格)"("Value"=w327) -> ()  [unwired: 2 in, 2 out]
                      n266 = Less?(x=w325, y=w328) -> (x < y?=w329:bool)
                    }
                    n267 = property on="强度图" class="IntGraph (严格)"() -> ("Value"=w285:dbl[][])  [unwired: 2 in, 2 out]
                    n268 = local read "Yloop"() -> (w296:dbl)
                    n269 = Decrement(x=w296) -> (x-1=w297:dbl)
                    n270 = local read "Y序"() -> (w283:i32)
                    n271 = Replace Array Subset(array=w285, new element=w284, index (col)=w283) -> (w286:dbl[][])  [unwired: 1 in]
                    n272 = property on="强度图" class="IntGraph (严格)"("Value"=w286) -> ()  [unwired: 2 in, 2 out]
                    n273 = Equal?(x=w283, y=w297) -> (x = y?=w303:bool)
                    n274 = Increment(x=w283) -> ()  [unwired: 1 out]
                    n275 = flat-sequence {
                      tunnel: w279 -> [w309]
                      tunnel: [w309] -> w278
                      frame #0 {
                        n276 = local read "毫秒计时值"() -> (w304:u32)
                        n277 = Tick Count (ms)() -> (millisecond timer value=w308:u32)
                        n278 = Subtract(x=w308, y=w304) -> (x-y=w305:u32)
                        n279 = Multiply(x=w305, y=0.001) -> (x*y=→"已用时（s）":dbl)
                      }
                    }
                    n280 = property on="细分设置" class="DigNum (严格)"() -> ("Value"=w289:dbl)  [unwired: 2 in, 2 out]
                    n281 = property on="等待时间" class="DigNum (严格)"() -> ("Value"=w290:u32)  [unwired: 2 in, 2 out]
                    n282 = case shown="假" w303 {
                      tunnel: w278 -> [w387 w419]
                      tunnel: [w385 w420] -> w301
                      tunnel: w290 -> [w383 w417]
                      tunnel: w289 -> [w382 w416]
                      frame False {
                        n283 = flat-sequence {
                          tunnel: w387 -> [w391]
                          tunnel: [w391] -> w386
                          tunnel: [w389] -> w384
                          tunnel: w383 -> [w390]
                          tunnel: w382 -> [w389]
                          frame #0 {
                            n284 = call "X,Y,Z轴坐标查询.vi"("细分设置"=w389, "查询坐标轴"="Y", "串口通信端口"=w391) -> ("坐标(mm)"=w392:dbl)
                            n285 = property on="Y:" class="DigNum (严格)"() -> ("Value"=w388:dbl)  [unwired: 2 in, 2 out]
                            n286 = Add(x=w392, y=w388) -> (x+y=w394:dbl)
                            "x+y 2" <- w394
                            n287 = Multiply(x=w394, y=200.0) -> (x*y=w398:dbl)
                            n288 = Multiply(x=w398, y=8.0 ("细分设置")) -> (x*y=w403:dbl)
                            n289 = Number To Fractional String(number=w403, precision (6)=i16 0 ("精度(6)")) -> (F-format string=w401:string)  [unwired: 2 out]
                            n290 = Concatenate Strings("Y=" ("字符串"), w401, "/" ("字符串")) -> (w396:string)
                            n291 = call "步进电机命令输入与输出.vi"("输入字符串"=w396, "串口通信端口"=w391) -> ()  [unwired: 1 out]
                            n292 = Wait (ms)(milliseconds to wait=w390) -> ()  [unwired: 1 out]
                          }
                        }
                        n293 = while {
                          shift-right: [w405] -> w385
                          shift-left: w386 -> [w405]
                          shift-right: [w404] -> _
                          shift-left: w384 -> [w404]
                          stop <- w411 stop-if-true
                          n294 = call "X,Y,Z轴坐标查询.vi"("细分设置"=w404, "查询坐标轴"="Y", "串口通信端口"=w405) -> ("坐标(mm)"=w409:dbl)
                          n295 = local read "x+y 2"() -> (w412:dbl)
                          n296 = property on="电机急停" class="Bool (严格)"() -> ("Value"=w408:bool)  [unwired: 2 in, 2 out]
                          n297 = property on="Y(mm)" class="DigNum (严格)"("Value"=w409) -> ()  [unwired: 2 in, 2 out]
                          n298 = case shown="真" w408 {
                            tunnel: w405 -> [_ w414]
                            frame False {
                            }
                            frame True {
                              n299 = call "步进电机命令输入与输出.vi"("输入字符串"="S0/", "串口通信端口"=w414) -> ()  [unwired: 1 out]
                            }
                          }
                          n300 = Subtract(x=w412, y=w409) -> (x-y=w407:dbl)
                          n301 = Absolute Value(x=w407) -> (abs(x)=w406:dbl)
                          n302 = local read "精度"() -> (w410:dbl)
                          n303 = Less?(x=w406, y=w410) -> (x < y?=w411:bool)
                        }
                      }
                      frame True {
                        n304 = flat-sequence {
                          tunnel: [w424] -> _
                          tunnel: [w424] -> w421
                          tunnel: w419 -> [w424]
                          tunnel: [w422] -> w418
                          tunnel: w417 -> [w423]
                          tunnel: w416 -> [w422]
                          frame #0 {
                            n305 = Multiply(x=0.0, y=200.0) -> (x*y=w428:dbl)
                            n306 = Multiply(x=w428, y=w422) -> (x*y=w433:dbl)
                            n307 = Number To Fractional String(number=w433, precision (6)=i16 0 ("精度(6)")) -> (F-format string=w431:string)  [unwired: 2 out]
                            n308 = Concatenate Strings("Y=" ("字符串"), w431, "/" ("字符串")) -> (w426:string)
                            n309 = call "步进电机命令输入与输出.vi"("输入字符串"=w426, "串口通信端口"=w424) -> ()  [unwired: 1 out]
                            n310 = Wait (ms)(milliseconds to wait=w423) -> ()  [unwired: 1 out]
                          }
                        }
                        n311 = while {
                          shift-right: [w435] -> w420
                          shift-left: w421 -> [w435]
                          shift-right: [w434] -> _
                          shift-left: w418 -> [w434]
                          stop <- w441 stop-if-true
                          n312 = property on="电机急停" class="Bool (严格)"() -> ("Value"=w442:bool)  [unwired: 2 in, 2 out]
                          n313 = call "X,Y,Z轴坐标查询.vi"("细分设置"=w434, "查询坐标轴"="Y", "串口通信端口"=w435) -> ("坐标(mm)"=w443:dbl)
                          n314 = case shown="真" w442 {
                            tunnel: w435 -> [_ w446]
                            frame False {
                            }
                            frame True {
                              n315 = call "步进电机命令输入与输出.vi"("输入字符串"="S0/", "串口通信端口"=w446) -> ()  [unwired: 1 out]
                            }
                          }
                          n316 = Multiply(x=w443, y=1.0 ("x")) -> (x*y=w439:dbl)
                          n317 = Subtract(x=w439, y=0.0 ("x")) -> (x-y=w437:dbl)
                          n318 = local read "精度"() -> (w440:dbl)
                          n319 = Absolute Value(x=w437) -> (abs(x)=w436:dbl)
                          n320 = property on="Y(mm)" class="DigNum (严格)"("Value"=w439) -> ()  [unwired: 2 in, 2 out]
                          n321 = Less?(x=w436, y=w440) -> (x < y?=w441:bool)
                        }
                      }
                    }
                    "Y序" <- w302
                  }
                  n322 = property on="已用时（s）" class="DigNum (严格)"("Visible"=TRUE ("可见")) -> ()  [unwired: 2 in, 2 out]
                  n323 = flat-sequence {
                    tunnel: [w227] -> w210
                    tunnel: ["文件保存"] -> w208
                    tunnel: w208 -> [w232]
                    tunnel: [w231] -> w207
                    frame #0 {
                      n324 = Build Path(base path="文件保存", name or relative path="频域谱" ("名称或相对路径")) -> (appended path=w230:path)
                      n325 = Create Folder(path (use dialog)=w230) -> (created path=w227:path)  [unwired: 2 in, 2 out]
                    }
                    frame #1 {
                      n326 = Build Path(base path=w232, name or relative path="时域谱" ("名称或相对路径")) -> (appended path=w233:path)
                      n327 = Create Folder(path (use dialog)=w233) -> (created path=w231:path)  [unwired: 2 in, 2 out]
                    }
                  }
                  n328 = flat-sequence {
                    tunnel: w222 -> [w237]
                    tunnel: [w235] -> _
                    tunnel: [w235] -> w204
                    tunnel: [w237] -> w203
                    tunnel: w202 -> [w235]
                    tunnel: [w238] -> w221
                    tunnel: w204 -> [w238]
                    tunnel: w203 -> [w241]
                    frame #0 {
                      n329 = property on="水平进度条" class="Slide (严格)"("Value"=u8 100 ("水平进度条")) -> ()  [unwired: 2 in, 2 out]
                    }
                    frame #1 {
                      n330 = local read "毫秒计时值"() -> (w240:u32)
                      n331 = Tick Count (ms)() -> (millisecond timer value=w245:u32)
                      n332 = Transpose 2D Array(2D array=w241) -> (transposed array=w242:dbl[][])
                      n333 = Subtract(x=w245, y=w240) -> (x-y=w243:u32)
                      n334 = property on="强度图" class="IntGraph (严格)"("Value"=w242) -> ()  [unwired: 2 in, 2 out]
                      n335 = Multiply(x=w243, y=0.001) -> (x*y=w239:dbl)
                      n336 = property on="已用时（s）" class="DigNum (严格)"("Value"=w239) -> ()  [unwired: 2 in, 2 out]
                      "数组" <- w241
                    }
                  }
                }
                event "逐行扫描": Value Change {
                  n337 = event-data() -> ()  [unwired: 1 in, 6 out]
                  n338 = flat-sequence {
                    tunnel: [w631] -> w544
                    tunnel: [w630] -> w541
                    tunnel: w544 -> [w635]
                    tunnel: [w634] -> w543
                    frame #0 {
                      n339 = local read "文件保存"() -> (w631:path)
                      n340 = Build Path(base path=w631, name or relative path="频域谱" ("名称或相对路径")) -> (appended path=w633:path)
                      n341 = Create Folder(path (use dialog)=w633) -> (created path=w630:path)  [unwired: 2 in, 2 out]
                    }
                    frame #1 {
                      n342 = Build Path(base path=w635, name or relative path="时域谱" ("名称或相对路径")) -> (appended path=w636:path)
                      n343 = Create Folder(path (use dialog)=w636) -> (created path=w634:path)  [unwired: 2 in, 2 out]
                    }
                  }
                  n344 = flat-sequence {
                    tunnel: [w588] -> w539
                    tunnel: w540 -> [w588]
                    frame #0 {
                      # "如果强度图那里出了错，就把这里的行列互换"
                      n345 = property on="Y起点" class="DigNum (严格)"() -> ("Value"=w591:dbl)  [unwired: 2 in, 2 out]
                      n346 = property on="细分设置" class="DigNum (严格)"() -> ("Value"=w589:dbl)  [unwired: 2 in, 2 out]
                      n347 = local read "Xloop"() -> (w595:dbl)
                      n348 = local read "Yloop"() -> (w594:dbl)
                      n349 = Multiply(x=w591, y=200.0) -> (x*y=w599:dbl)
                      n350 = Tick Count (ms)() -> (millisecond timer value=w592:u32)
                      n351 = Multiply(x=w599, y=w589) -> (x*y=w604:dbl)
                      n352 = Initialize Array(0.0 ("元素"), w595, w594) -> (w590:dbl[][])
                      n353 = Number To Fractional String(number=w604, precision (6)=i16 0 ("精度(6)")) -> (F-format string=w602:string)  [unwired: 2 out]
                      n354 = property on="毫秒计时值" class="DigNum (严格)"("Value"=w592) -> ()  [unwired: 2 in, 2 out]
                      n355 = property on="强度图" class="IntGraph (严格)"("Value"=w590) -> ()  [unwired: 2 in, 2 out]
                      n356 = Concatenate Strings("Y=" ("字符串"), w602, "/" ("字符串")) -> (w597:string)
                      n357 = call "步进电机命令输入与输出.vi"("输入字符串"=w597, "串口通信端口"=w588) -> ()  [unwired: 1 out]
                      n358 = property on="等待时间" class="DigNum (严格)"() -> ("Value"=w593:u32)  [unwired: 2 in, 2 out]
                      n359 = property on="已用时（s）" class="DigNum (严格)"("Value"=0.0 ("已用时（s）")) -> ()  [unwired: 2 in, 2 out]
                      n360 = Wait (ms)(milliseconds to wait=w593) -> ()  [unwired: 1 out]
                    }
                  }
                  n361 = property on="水平进度条" class="Slide (严格)"("Visible"=TRUE ("可见")) -> ()  [unwired: 2 in, 2 out]
                  n362 = property on="单行？" class="RadioBtnsControl (严格)"("Visible"=FALSE ("可见")) -> ()  [unwired: 2 in, 2 out]
                  n363 = flat-sequence {
                    tunnel: [w583] -> w538
                    frame #0 {
                      n364 = property on="X终点" class="DigNum (严格)"() -> ("Value"=w572:dbl)  [unwired: 2 in, 2 out]
                      n365 = property on="X起点" class="DigNum (严格)"() -> ("Value"=w571:dbl)  [unwired: 2 in, 2 out]
                      n366 = Subtract(x=w572, y=w571) -> (x-y=w576:dbl)
                      n367 = local read "X:"() -> (w575:dbl)
                      n368 = property on="X扫描范围" class="DigNum (严格)"("Value"=w576) -> ()  [unwired: 2 in, 2 out]
                      n369 = Divide(x=w576, y=w575) -> (x/y=w574:dbl)
                      n370 = Increment(x=w574) -> (x+1=w573:dbl)
                      n371 = property on="Xloop" class="DigNum (严格)"("Value"=w573) -> ()  [unwired: 2 in, 2 out]
                    }
                    frame #1 {
                      n372 = property on="Y终点" class="DigNum (严格)"() -> ("Value"=w578:dbl)  [unwired: 2 in, 2 out]
                      n373 = property on="Y起点" class="DigNum (严格)"() -> ("Value"=w577:dbl)  [unwired: 2 in, 2 out]
                      n374 = Subtract(x=w578, y=w577) -> (x-y=w581:dbl)
                      n375 = local read "Y:"() -> (w580:dbl)
                      n376 = property on="Y扫描范围" class="DigNum (严格)"("Value"=w581) -> ()  [unwired: 2 in, 2 out]
                      n377 = Divide(x=w581, y=w580) -> (x/y=w582:dbl)
                      n378 = Increment(x=w582) -> (x+1=w579:dbl)
                      n379 = property on="Yloop" class="DigNum (严格)"("Value"=w579) -> ()  [unwired: 2 in, 2 out]
                    }
                    frame #2 {
                      n380 = property on="Xloop" class="DigNum (严格)"() -> ("Value"=w586:dbl)  [unwired: 2 in, 2 out]
                      n381 = property on="Yloop" class="DigNum (严格)"() -> ("Value"=w583:dbl)  [unwired: 2 in, 2 out]
                      n382 = Initialize Array(0.0 ("元素"), w586, w583) -> (w585:dbl[][])
                      n383 = property on="强度图" class="IntGraph (严格)"("Value"=w585) -> ()  [unwired: 2 in, 2 out]
                    }
                  }
                  n384 = while {
                    shift-right: [w606] -> w528
                    shift-left: w539 -> [w606]
                    stop <- w611 stop-if-true
                    n385 = call "X,Y,Z轴坐标查询.vi"("细分设置"=8.0, "查询坐标轴"="Y", "串口通信端口"=w606) -> ("坐标(mm)"=w613:dbl)
                    n386 = property on="Y起点" class="DigNum (严格)"() -> ("Value"=w605:dbl)  [unwired: 2 in, 2 out]
                    n387 = property on="电机急停" class="Bool (严格)"() -> ("Value"=w612:bool)  [unwired: 2 in, 2 out]
                    n388 = Multiply(x=w613, y=1.0 ("x")) -> (x*y=w609:dbl)
                    n389 = Subtract(x=w605, y=w609) -> (x-y=w608:dbl)
                    n390 = case shown="真" w612 {
                      tunnel: w606 -> [_ w617]
                      frame False {
                      }
                      frame True {
                        n391 = call "步进电机命令输入与输出.vi"("输入字符串"="S0/", "串口通信端口"=w617) -> ()  [unwired: 1 out]
                      }
                    }
                    n392 = Absolute Value(x=w608) -> (abs(x)=w607:dbl)
                    n393 = local read "精度"() -> (w610:dbl)
                    n394 = property on="Y(mm)" class="DigNum (严格)"("Value"=w609) -> ()  [unwired: 2 in, 2 out]
                    n395 = Less?(x=w607, y=w610) -> (x < y?=w611:bool)
                  }
                  n396 = flat-sequence {
                    tunnel: w528 -> [w548]
                    tunnel: [w548] -> w530
                    tunnel: [w545] -> w529
                    frame #0 {
                      n397 = property on="细分设置" class="DigNum (严格)"() -> ("Value"=w545:dbl)  [unwired: 2 in, 2 out]
                      n398 = Multiply(x=0.0, y=50.0) -> (x*y=w551:dbl)
                      n399 = Multiply(x=w551, y=w545) -> (x*y=w556:dbl)
                      n400 = Number To Fractional String(number=w556, precision (6)=i16 0 ("精度(6)")) -> (F-format string=w554:string)  [unwired: 2 out]
                      n401 = Concatenate Strings("X=" ("字符串"), w554, "/" ("字符串")) -> (w549:string)
                      n402 = call "步进电机命令输入与输出.vi"("输入字符串"=w549, "串口通信端口"=w548) -> ()  [unwired: 1 out]
                      n403 = property on="等待时间" class="DigNum (严格)"() -> ("Value"=w546:u32)  [unwired: 2 in, 2 out]
                      n404 = Wait (ms)(milliseconds to wait=w546) -> ()  [unwired: 1 out]
                    }
                  }
                  n405 = while {
                    shift-right: [w558] -> w527
                    shift-left: w530 -> [w558]
                    shift-right: [w557] -> _
                    shift-left: w529 -> [w557]
                    stop <- w564 stop-if-true
                    n406 = property on="电机急停" class="Bool (严格)"() -> ("Value"=w565:bool)  [unwired: 2 in, 2 out]
                    n407 = call "X,Y,Z轴坐标查询.vi"("细分设置"=w557, "查询坐标轴"="X", "串口通信端口"=w558) -> ("坐标(mm)"=w566:dbl)
                    n408 = case shown="真" w565 {
                      tunnel: w558 -> [_ w569]
                      frame False {
                      }
                      frame True {
                        n409 = call "步进电机命令输入与输出.vi"("输入字符串"="S0/", "串口通信端口"=w569) -> ()  [unwired: 1 out]
                      }
                    }
                    n410 = Multiply(x=w566, y=4.0 ("x")) -> (x*y=w562:dbl)
                    n411 = Subtract(x=0.0, y=w562) -> (x-y=w561:dbl)
                    n412 = Absolute Value(x=w561) -> (abs(x)=w560:dbl)
                    n413 = local read "精度"() -> (w563:dbl)
                    n414 = property on="X（mm）" class="DigNum (严格)"("Value"=w562) -> ()  [unwired: 2 in, 2 out]
                    n415 = Less?(x=w560, y=w563) -> (x < y?=w564:bool)
                  }
                  n416 = for {
                    N: w538 -> [_]
                    shift-right: [w653] -> _
                    shift-left: w541 -> [w653]
                    shift-right: [w652] -> _
                    shift-left: w543 -> [w652]
                    tunnel: [w651] -> w537 mode=indexing
                    shift-right: [w644] -> w536
                    shift-left: w527 -> [w646]
                    i -> [w639]
                    # "实时成像出问题调这里"
                    n417 = local read "Yloop"() -> (w641:dbl)
                    n418 = property on="Y序" class="DigNum (严格)"("Value"=w639) -> ()  [unwired: 2 in, 2 out]
                    n419 = Multiply(x=w641, y=0.01) -> (x*y=w640:dbl)
                    n420 = Divide(x=w639, y=w640) -> (x/y=w642:dbl)
                    n421 = property on="水平进度条" class="Slide (严格)"("Value"=w642) -> ()  [unwired: 2 in, 2 out]
                    n422 = case shown="\"双行\"" "单行？" {
                      tunnel: w653 -> [w664 w739]
                      tunnel: w652 -> [w663 w740]
                      tunnel: [w662 w736] -> w651
                      tunnel: [w658 w734] -> w649
                      tunnel: w646 -> [w657 w738]
                      frame "单行", Default {
                        n423 = flat-sequence {
                          tunnel: [w698] -> w667
                          tunnel: [w696] -> w666
                          tunnel: [w699] -> w662
                          tunnel: [w697] -> w665
                          tunnel: w657 -> [w695]
                          tunnel: [w729] -> w659
                          tunnel: w663 -> [w713]
                          tunnel: w664 -> [w712]
                          tunnel: w667 -> [w725]
                          tunnel: w666 -> [w729]
                          tunnel: w665 -> [w717]
                          frame #0 {
                            n424 = local read "精度"() -> (w707:dbl)
                            n425 = property on="细分设置" class="DigNum (严格)"() -> ("Value"=w706:dbl)  [unwired: 2 in, 2 out]
                            n426 = property on="X终点" class="DigNum (严格)"() -> ("Value"=w710:dbl)  [unwired: 2 in, 2 out]
                            n427 = property on="X起点" class="DigNum (严格)"() -> ("Value"=w694:dbl)  [unwired: 2 in, 2 out]
                            n428 = local read item#-1() -> (w702)
                            n429 = local read item#-1() -> (w704)
                            n430 = property on="等待时间" class="DigNum (严格)"() -> ("Value"=w708:u32)  [unwired: 2 in, 2 out]
                            n431 = property on="电机急停" class="Bool (严格)"() -> ("Value"=w709:bool)  [unwired: 2 in, 2 out]
                            n432 = call "X轴连续扫描（1.0）.vi"("VISA I"=w695, "X0"=w694, "X"=w710, "精度"=w707, "细分设置"=w706, "等待时间(ms)"=w708, "pulDDR2Length"=w702, "电机急停"=w709, "M-length"=w704) -> ("hDevice"=w703:i32, "N-length"=w705:dbl, "VISA O"=w696:refnum<visa-resource-name>, "hDevice out"=w701:i32, "X"=w700:dbl, "强度图行"=w699:dbl[], "时域谱页"=w698:dbl[][], "幅频谱页"=w697:dbl[][])  [unwired: 3 in]
                            n433 = property on="hDevice 2" class="DigNum (严格)"("Value"=w701) -> ()  [unwired: 2 in, 2 out]
                            n434 = property on="X（mm）" class="DigNum (严格)"("Value"=w700) -> ()  [unwired: 2 in, 2 out]
                          }
                          frame #1 {
                            n435 = property on="Y序" class="DigNum (严格)"() -> ("Value"=w711:i32)  [unwired: 2 in, 2 out]
                            n436 = Increment(x=w711) -> (x+1=w714:i32)
                            n437 = Number To Decimal String(number=w714) -> (decimal integer string=w723:string)  [unwired: 1 in]
                            n438 = Number To Decimal String(number=w714) -> (decimal integer string=w722:string)  [unwired: 1 in]
                            n439 = Concatenate Strings("T" ("字符串"), w723, ".txt" ("字符串")) -> (w726:string)
                            n440 = Concatenate Strings("F" ("字符串"), w722, ".txt" ("字符串")) -> (w720:string)
                            n441 = Build Path(base path=w713, name or relative path=w726) -> (appended path=w728:path)
                            n442 = call-poly <vilib>:"Write Delimited Spreadsheet.vi"("file path (dialog if empty)"=w728, "2D data"=w725, "transpose? (no:F)"=FALSE) -> ()  [unwired: 11 in, 2 out]
                            n443 = Build Path(base path=w712, name or relative path=w720) -> (appended path=w718:path)
                            n444 = call-poly <vilib>:"Write Delimited Spreadsheet.vi"("file path (dialog if empty)"=w718, "2D data"=w717, "transpose? (no:F)"=FALSE) -> ()  [unwired: 11 in, 2 out]
                          }
                        }
                        n445 = flat-sequence {
                          tunnel: w659 -> [w671]
                          tunnel: [w671] -> w660
                          tunnel: [w670] -> w661
                          frame #0 {
                            n446 = property on="细分设置" class="DigNum (严格)"() -> ("Value"=w670:dbl)  [unwired: 2 in, 2 out]
                            n447 = Multiply(x=0.0, y=50.0) -> (x*y=w674:dbl)
                            n448 = Multiply(x=w674, y=w670) -> (x*y=w679:dbl)
                            n449 = local read "等待时间"() -> (w669:u32)
                            n450 = Number To Fractional String(number=w679, precision (6)=i16 0 ("精度(6)")) -> (F-format string=w677:string)  [unwired: 2 out]
                            n451 = Concatenate Strings("X=" ("字符串"), w677, "/" ("字符串")) -> (w672:string)
                            n452 = Wait (ms)(milliseconds to wait=w669) -> ()  [unwired: 1 out]
                            n453 = call "步进电机命令输入与输出.vi"("输入字符串"=w672, "串口通信端口"=w671) -> ()  [unwired: 1 out]
                          }
                        }
                        n454 = while {
                          shift-right: [w683] -> w658
                          shift-left: w660 -> [w683]
                          shift-right: [w681] -> _
                          shift-left: w661 -> [w681]
                          stop <- w687 stop-if-true
                          n455 = property on="电机急停" class="Bool (严格)"() -> ("Value"=w688:bool)  [unwired: 2 in, 2 out]
                          n456 = case shown="真" w688 {
                            tunnel: w683 -> [_ w692]
                            frame False {
                            }
                            frame True {
                              n457 = call "步进电机命令输入与输出.vi"("输入字符串"="S0/", "串口通信端口"=w692) -> ()  [unwired: 1 out]
                            }
                          }
                          n458 = call "X,Y,Z轴坐标查询.vi"("细分设置"=w681, "查询坐标轴"="X", "串口通信端口"=w683) -> ("坐标(mm)"=w689:dbl)
                          n459 = Multiply(x=w689, y=4.0 ("x")) -> (x*y=w685:dbl)
                          n460 = Subtract(x=0.0, y=w685) -> (x-y=w684:dbl)
                          n461 = local read "精度"() -> (w686:dbl)
                          n462 = Absolute Value(x=w684) -> (abs(x)=w682:dbl)
                          n463 = property on="X（mm）" class="DigNum (严格)"("Value"=w685) -> ()  [unwired: 2 in, 2 out]
                          n464 = Less?(x=w682, y=w686) -> (x < y?=w687:bool)
                        }
                      }
                      frame "双行" {
                        n465 = flat-sequence {
                          tunnel: [w781] -> w743
                          tunnel: [w779] -> w742
                          tunnel: [w782] -> w736
                          tunnel: [w780] -> w741
                          tunnel: w738 -> [w778]
                          tunnel: [w775] -> w737
                          tunnel: [w835] -> w735
                          tunnel: w740 -> [w819]
                          tunnel: w739 -> [w818]
                          tunnel: w743 -> [w831]
                          tunnel: w742 -> [w835]
                          tunnel: w741 -> [w823]
                          tunnel: w737 -> [w817]
                          tunnel: [w817] -> w730
                          frame #0 {
                            n466 = property on="Y序" class="DigNum (严格)"() -> ("Value"=w775:i32)  [unwired: 2 in, 2 out]
                            n467 = Power Of X(1:-1.0 ("x"), 2:w775) -> (0:w776:dbl)
                            n468 = case shown="-1" w776 {
                              tunnel: [w786 w807] -> w782
                              tunnel: [w789 w806] -> w781
                              tunnel: [w788 w805] -> w780
                              tunnel: [w787 w804] -> w779
                              tunnel: w778 -> [w785 w803]
                              frame -1 {
                                n469 = local read "精度"() -> (w796:dbl)
                                n470 = property on="细分设置" class="DigNum (严格)"() -> ("Value"=w795:dbl)  [unwired: 2 in, 2 out]
                                n471 = property on="X终点" class="DigNum (严格)"() -> ("Value"=w799:dbl)  [unwired: 2 in, 2 out]
                                n472 = property on="X起点" class="DigNum (严格)"() -> ("Value"=w790:dbl)  [unwired: 2 in, 2 out]
                                n473 = local read "量程选择 0"() -> (w793:i32)
                                n474 = local read "触发输出"() -> (w794:i32)
                                n475 = property on="等待时间" class="DigNum (严格)"() -> ("Value"=w797:u32)  [unwired: 2 in, 2 out]
                                n476 = property on="电机急停" class="Bool (严格)"() -> ("Value"=w798:bool)  [unwired: 2 in, 2 out]
                                n477 = call "X轴回程连续扫描（1.0）.vi"("VISA I"=w785, "X0"=w790, "X"=w799, "精度"=w796, "细分设置"=w795, "等待时间(ms)"=w797, "pulDDR2Length"=w793, "电机急停"=w798, "M-length"=w794, "N-length"="输出宽度 2") -> ("hDevice"=w784:i32, "VISA O"=w787:refnum<visa-resource-name>, "hDevice out"=w792:i32, "X"=w791:dbl, "强度图行"=w786:dbl[], "时域谱页"=w789:dbl[][], "幅频谱页"=w788:dbl[][])  [unwired: 3 in]
                                n478 = property on="X（mm）" class="DigNum (严格)"("Value"=w791) -> ()  [unwired: 2 in, 2 out]
                                n479 = property on="hDevice 2" class="DigNum (严格)"("Value"=w792) -> ()  [unwired: 2 in, 2 out]
                              }
                              frame 1, Default {
                                n480 = local read "精度"() -> (w813:dbl)
                                n481 = property on="细分设置" class="DigNum (严格)"() -> ("Value"=w812:dbl)  [unwired: 2 in, 2 out]
                                n482 = property on="X终点" class="DigNum (严格)"() -> ("Value"=w816:dbl)  [unwired: 2 in, 2 out]
                                n483 = property on="X起点" class="DigNum (严格)"() -> ("Value"=w802:dbl)  [unwired: 2 in, 2 out]
                                n484 = local read "量程选择 0"() -> (w810:i32)
                                n485 = local read "触发输出"() -> (w811:i32)
                                n486 = property on="等待时间" class="DigNum (严格)"() -> ("Value"=w814:u32)  [unwired: 2 in, 2 out]
                                n487 = property on="电机急停" class="Bool (严格)"() -> ("Value"=w815:bool)  [unwired: 2 in, 2 out]
                                n488 = call "X轴连续扫描（1.0）.vi"("VISA I"=w803, "X0"=w802, "X"=w816, "精度"=w813, "细分设置"=w812, "等待时间(ms)"=w814, "pulDDR2Length"=w810, "电机急停"=w815, "M-length"=w811, "N-length"="输出宽度 3") -> ("hDevice"=w800:i32, "VISA O"=w804:refnum<visa-resource-name>, "hDevice out"=w809:i32, "X"=w808:dbl, "强度图行"=w807:dbl[], "时域谱页"=w806:dbl[][], "幅频谱页"=w805:dbl[][])  [unwired: 3 in]
                                n489 = property on="hDevice 2" class="DigNum (严格)"("Value"=w809) -> ()  [unwired: 2 in, 2 out]
                                n490 = property on="X（mm）" class="DigNum (严格)"("Value"=w808) -> ()  [unwired: 2 in, 2 out]
                              }
                            }
                          }
                          frame #1 {
                            n491 = Increment(x=w817) -> (x+1=w820:i32)
                            n492 = Number To Decimal String(number=w820) -> (decimal integer string=w829:string)  [unwired: 1 in]
                            n493 = Number To Decimal String(number=w820) -> (decimal integer string=w828:string)  [unwired: 1 in]
                            n494 = Concatenate Strings("T" ("字符串"), w829, ".txt" ("字符串")) -> (w832:string)
                            n495 = Concatenate Strings("F" ("字符串"), w828, ".txt" ("字符串")) -> (w826:string)
                            n496 = Build Path(base path=w819, name or relative path=w832) -> (appended path=w834:path)
                            n497 = call-poly <vilib>:"Write Delimited Spreadsheet.vi"("file path (dialog if empty)"=w834, "2D data"=w831, "transpose? (no:F)"=FALSE) -> ()  [unwired: 11 in, 2 out]
                            n498 = Build Path(base path=w818, name or relative path=w826) -> (appended path=w824:path)
                            n499 = call-poly <vilib>:"Write Delimited Spreadsheet.vi"("file path (dialog if empty)"=w824, "2D data"=w823, "transpose? (no:F)"=FALSE) -> ()  [unwired: 11 in, 2 out]
                          }
                        }
                        n500 = property on="Yloop" class="DigNum (严格)"() -> ("Value"=w733:dbl)  [unwired: 2 in, 2 out]
                        n501 = Decrement(x=w733) -> (x-1=w732:dbl)
                        n502 = Equal?(x=w730, y=w732) -> (x = y?=w731:bool)
                        n503 = case shown="假" w731 {
                          tunnel: w735 -> [w744 w745]
                          tunnel: [w744 w746] -> w734
                          frame False {
                          }
                          frame True {
                            n504 = flat-sequence {
                              tunnel: w745 -> [w752]
                              tunnel: [w752] -> w747
                              tunnel: [w751] -> w748
                              frame #0 {
                                n505 = property on="细分设置" class="DigNum (严格)"() -> ("Value"=w751:dbl)  [unwired: 2 in, 2 out]
                                n506 = Multiply(x=0.0, y=50.0) -> (x*y=w755:dbl)
                                n507 = Multiply(x=w755, y=w751) -> (x*y=w760:dbl)
                                n508 = local read "等待时间"() -> (w750:u32)
                                n509 = Number To Fractional String(number=w760, precision (6)=i16 0 ("精度(6)")) -> (F-format string=w758:string)  [unwired: 2 out]
                                n510 = Concatenate Strings("X=" ("字符串"), w758, "/" ("字符串")) -> (w753:string)
                                n511 = Wait (ms)(milliseconds to wait=w750) -> ()  [unwired: 1 out]
                                n512 = call "步进电机命令输入与输出.vi"("输入字符串"=w753, "串口通信端口"=w752) -> ()  [unwired: 1 out]
                              }
                            }
                            n513 = while {
                              shift-right: [w764] -> w746
                              shift-left: w747 -> [w764]
                              shift-right: [w762] -> _
                              shift-left: w748 -> [w762]
                              stop <- w768 stop-if-true
                              n514 = property on="电机急停" class="Bool (严格)"() -> ("Value"=w769:bool)  [unwired: 2 in, 2 out]
                              n515 = case shown="真" w769 {
                                tunnel: w764 -> [_ w773]
                                frame False {
                                }
                                frame True {
                                n516 = call "步进电机命令输入与输出.vi"("输入字符串"="S0/", "串口通信端口"=w773) -> ()  [unwired: 1 out]
                                }
                              }
                              n517 = call "X,Y,Z轴坐标查询.vi"("细分设置"=w762, "查询坐标轴"="X", "串口通信端口"=w764) -> ("坐标(mm)"=w770:dbl)
                              n518 = Multiply(x=w770, y=4.0 ("x")) -> (x*y=w766:dbl)
                              n519 = Subtract(x=0.0, y=w766) -> (x-y=w765:dbl)
                              n520 = local read "精度"() -> (w767:dbl)
                              n521 = Absolute Value(x=w765) -> (abs(x)=w763:dbl)
                              n522 = property on="X（mm）" class="DigNum (严格)"("Value"=w766) -> ()  [unwired: 2 in, 2 out]
                              n523 = Less?(x=w763, y=w767) -> (x < y?=w768:bool)
                            }
                          }
                        }
                      }
                    }
                    n524 = property on="强度图" class="IntGraph (严格)"() -> ("Value"=w656:dbl[][])  [unwired: 2 in, 2 out]
                    n525 = property on="Yloop" class="DigNum (严格)"() -> ("Value"=w647:dbl)  [unwired: 2 in, 2 out]
                    n526 = property on="Y序" class="DigNum (严格)"() -> ("Value"=w650:i32)  [unwired: 2 in, 2 out]
                    n527 = Replace Array Subset(array=w656, new element=w651, index (col)=w650) -> (w655:dbl[][])  [unwired: 1 in]
                    n528 = property on="强度图" class="IntGraph (严格)"("Value"=w655) -> ()  [unwired: 2 in, 2 out]
                    n529 = Decrement(x=w647) -> (x-1=w648:dbl)
                    n530 = Equal?(x=w650, y=w648) -> (x = y?=w654:bool)
                    n531 = case shown="真" w654 {
                      tunnel: w649 -> [w845 w875]
                      tunnel: [w843 w876] -> w645
                      frame False {
                        n532 = flat-sequence {
                          tunnel: w845 -> [w849]
                          tunnel: [w849] -> w844
                          tunnel: [w846] -> w842
                          frame #0 {
                            n533 = property on="细分设置" class="DigNum (严格)"() -> ("Value"=w846:dbl)  [unwired: 2 in, 2 out]
                            n534 = call "X,Y,Z轴坐标查询.vi"("细分设置"=w846, "查询坐标轴"="Y", "串口通信端口"=w849) -> ("坐标(mm)"=w850:dbl)
                            n535 = property on="Y:" class="DigNum (严格)"() -> ("Value"=w848:dbl)  [unwired: 2 in, 2 out]
                            n536 = Add(x=w850, y=w848) -> (x+y=w852:dbl)
                            "x+y 3" <- w852
                            n537 = Multiply(x=w852, y=200.0) -> (x*y=w856:dbl)
                            n538 = Multiply(x=w856, y=8.0 ("细分设置")) -> (x*y=w861:dbl)
                            n539 = Number To Fractional String(number=w861, precision (6)=i16 0 ("精度(6)")) -> (F-format string=w859:string)  [unwired: 2 out]
                            n540 = Concatenate Strings("Y=" ("字符串"), w859, "/" ("字符串")) -> (w854:string)
                            n541 = call "步进电机命令输入与输出.vi"("输入字符串"=w854, "串口通信端口"=w849) -> ()  [unwired: 1 out]
                            n542 = property on="等待时间" class="DigNum (严格)"() -> ("Value"=w847:u32)  [unwired: 2 in, 2 out]
                            n543 = Wait (ms)(milliseconds to wait=w847) -> ()  [unwired: 1 out]
                          }
                        }
                        n544 = while {
                          shift-right: [w864] -> w843
                          shift-left: w844 -> [w864]
                          shift-right: [w863] -> _
                          shift-left: w842 -> [w863]
                          stop <- w870 stop-if-true
                          n545 = call "X,Y,Z轴坐标查询.vi"("细分设置"=w863, "查询坐标轴"="Y", "串口通信端口"=w864) -> ("坐标(mm)"=w868:dbl)
                          n546 = property on="x+y 3" class="DigNum (严格)"() -> ("Value"=w862:dbl)  [unwired: 2 in, 2 out]
                          n547 = property on="电机急停" class="Bool (严格)"() -> ("Value"=w867:bool)  [unwired: 2 in, 2 out]
                          n548 = property on="Y(mm)" class="DigNum (严格)"("Value"=w868) -> ()  [unwired: 2 in, 2 out]
                          n549 = case shown="真" w867 {
                            tunnel: w864 -> [_ w872]
                            frame False {
                            }
                            frame True {
                              n550 = call "步进电机命令输入与输出.vi"("输入字符串"="S0/", "串口通信端口"=w872) -> ()  [unwired: 1 out]
                            }
                          }
                          n551 = Subtract(x=w862, y=w868) -> (x-y=w866:dbl)
                          n552 = Absolute Value(x=w866) -> (abs(x)=w865:dbl)
                          n553 = local read "精度"() -> (w869:dbl)
                          n554 = Less?(x=w865, y=w869) -> (x < y?=w870:bool)
                        }
                      }
                      frame True {
                        n555 = flat-sequence {
                          tunnel: [w880] -> _
                          tunnel: [w880] -> w877
                          tunnel: w875 -> [w880]
                          tunnel: [w878] -> w874
                          frame #0 {
                            n556 = property on="细分设置" class="DigNum (严格)"() -> ("Value"=w878:dbl)  [unwired: 2 in, 2 out]
                            n557 = Multiply(x=0.0, y=200.0) -> (x*y=w884:dbl)
                            n558 = Multiply(x=w884, y=w878) -> (x*y=w889:dbl)
                            n559 = Number To Fractional String(number=w889, precision (6)=i16 0 ("精度(6)")) -> (F-format string=w887:string)  [unwired: 2 out]
                            n560 = Concatenate Strings("Y=" ("字符串"), w887, "/" ("字符串")) -> (w882:string)
                            n561 = call "步进电机命令输入与输出.vi"("输入字符串"=w882, "串口通信端口"=w880) -> ()  [unwired: 1 out]
                            n562 = property on="等待时间" class="DigNum (严格)"() -> ("Value"=w879:u32)  [unwired: 2 in, 2 out]
                            n563 = Wait (ms)(milliseconds to wait=w879) -> ()  [unwired: 1 out]
                          }
                        }
                        n564 = while {
                          shift-right: [w891] -> w876
                          shift-left: w877 -> [w891]
                          shift-right: [w890] -> _
                          shift-left: w874 -> [w890]
                          stop <- w897 stop-if-true
                          n565 = property on="电机急停" class="Bool (严格)"() -> ("Value"=w898:bool)  [unwired: 2 in, 2 out]
                          n566 = call "X,Y,Z轴坐标查询.vi"("细分设置"=w890, "查询坐标轴"="Y", "串口通信端口"=w891) -> ("坐标(mm)"=w899:dbl)
                          n567 = case shown="真" w898 {
                            tunnel: w891 -> [_ w902]
                            frame False {
                            }
                            frame True {
                              n568 = call "步进电机命令输入与输出.vi"("输入字符串"="S0/", "串口通信端口"=w902) -> ()  [unwired: 1 out]
                            }
                          }
                          n569 = Multiply(x=w899, y=1.0 ("x")) -> (x*y=w895:dbl)
                          n570 = Subtract(x=w895, y=0.0 ("x")) -> (x-y=w893:dbl)
                          n571 = local read "精度"() -> (w896:dbl)
                          n572 = Absolute Value(x=w893) -> (abs(x)=w892:dbl)
                          n573 = property on="Y(mm)" class="DigNum (严格)"("Value"=w895) -> ()  [unwired: 2 in, 2 out]
                          n574 = Less?(x=w892, y=w896) -> (x < y?=w897:bool)
                        }
                      }
                    }
                    n575 = flat-sequence {
                      tunnel: w645 -> [w836]
                      tunnel: [w836] -> w644
                      frame #0 {
                        n576 = local read "毫秒计时值"() -> (w837:u32)
                        n577 = Tick Count (ms)() -> (millisecond timer value=w840:u32)
                        n578 = Subtract(x=w840, y=w837) -> (x-y=w838:u32)
                        n579 = Multiply(x=w838, y=0.001) -> (x*y=w841:dbl)
                        n580 = property on="已用时（s）" class="DigNum (严格)"("Value"=w841) -> ()  [unwired: 2 in, 2 out]
                      }
                    }
                  }
                  n581 = property on="已用时（s）" class="DigNum (严格)"("Visible"=TRUE ("可见")) -> ()  [unwired: 2 in, 2 out]
                  n582 = flat-sequence {
                    tunnel: w537 -> [w620]
                    tunnel: w536 -> [w621]
                    tunnel: [w621] -> w533
                    tunnel: [w620] -> w532
                    tunnel: [w623] -> w542
                    tunnel: w533 -> [w623]
                    tunnel: w532 -> [w624]
                    frame #0 {
                      n583 = property on="水平进度条" class="Slide (严格)"("Value"=u8 100 ("水平进度条")) -> ()  [unwired: 2 in, 2 out]
                    }
                    frame #1 {
                      n584 = local read "毫秒计时值"() -> (w628:u32)
                      n585 = property on="数组" class="Arr (严格)"("Value"=w624) -> ()  [unwired: 2 in, 2 out]
                      n586 = Transpose 2D Array(2D array=w624) -> (transposed array=w625:dbl[][])
                      n587 = Tick Count (ms)() -> (millisecond timer value=w629:u32)
                      n588 = property on="强度图" class="IntGraph (严格)"("Value"=w625) -> ()  [unwired: 2 in, 2 out]
                      n589 = Subtract(x=w629, y=w628) -> (x-y=w626:u32)
                      n590 = Multiply(x=w626, y=0.001) -> (x*y=w622:dbl)
                      n591 = property on="已用时（s）" class="DigNum (严格)"("Value"=w622) -> ()  [unwired: 2 in, 2 out]
                    }
                  }
                }
                event "分层图查看": Value Change {
                  n592 = event-data() -> ()  [unwired: 1 in, 6 out]
                  n593 = call "分层图显示1.2.1（导入色码表）.vi"("IN"=w905) -> ("OUT"=w904:string)  [unwired: 10 in]
                }
              }
            }
          }
        }
        n594 = dll-call lib="E:/PCI8552B/Driver/INF/Win32&Win64/amd64/PCI8552B_32.dll" fn="PCI8552B_StopDeviceAD" label="StopDeviceAD"("hDevice"="hDevice 2") -> ("hDevice"=w67:i32)  [unwired: 4 in, 2 out]
        n595 = dll-call lib="E:/PCI8552B/Driver/INF/Win32&Win64/amd64/PCI8552B_32.DLL" fn="PCI8552B_ReleaseDeviceAD" label="ReleaseDeviceAD"("hDevice"=w67) -> ("hDevice"=w66:i32)  [unwired: 4 in, 2 out]
        n596 = VISA Close(VISA resource name=w73) -> (error out=→"错误输出":errorcluster)  [unwired: 1 in]
        n597 = dll-call lib="E:/PCI8552B/Driver/INF/Win32&Win64/amd64/PCI8552B_32.DLL" fn="PCI8552B_ReleaseDevice" label="ReleaseDevice"("hDevice"=w66) -> ()  [unwired: 5 in, 2 out]
      }
    }
  }
  n598 = property on="高级设置" class="Bool"("Visible"=FALSE ("可见")) -> ()  [unwired: 2 in, 2 out]
  n599 = property on="定位模式" class="Bool"("Visible"=FALSE ("可见")) -> ()  [unwired: 2 in, 2 out]
  n600 = property on="已用时（s）" class="DigNum (严格)"("Visible"=FALSE ("可见")) -> ()  [unwired: 2 in, 2 out]
